vi "Run.vi"(8 "error in (no error)":errorcluster, 11 "Channel in":refnum<class "Channel.lvclass">) -> (0 "error out":errorcluster, 3 "Channel out":refnum<class "Channel.lvclass">)   [LabVIEW 2018, in "Channel.lvclass"]
uses:
  Channel.lvclass
  Channel.lvclass/Channel.ctl
  Simulated_CCD_Camera/Simulated_CCD_Camera.lvclass/Simulated_CCD_Camera.ctl
  State Machine/State Machine.lvclass/State Machine.ctl
  Save Image/Save Image.lvclass/Save Image.ctl
  Interface/Interface.lvclass/Interface.ctl
  Interface/Interface.lvclass
  State Machine/State Machine.lvclass
  Simulated_CCD_Camera/Simulated_CCD_Camera.lvclass
  Save Image/Save Image.lvclass
  RxTx/RxTx.lvclass
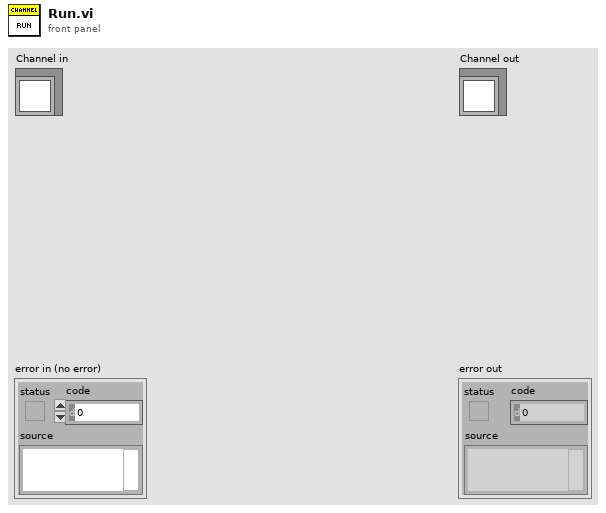
[diagram p1: front panel]
types:
  T1 = cluster{"PREAMP":u16, "READOUT_RATE":u16, "EM_GAIN":u16, "VBIN":u16, "INITIAL_LINE":u16, "INITIAL_COLUMN":u16, "FINAL_LINE":u16, "FINAL_COLUMN":u16, "TRIGGER_MODE":u16, "HBIN":u16, "SHUTTER_TTL":u16, "SHUTTER_MODE":u16, "SHUTTER_OPENING_TIME":u16, "SHUTTER_CLOSING_TIME":u16, "VERTICAL_SHIFT_SPEED":u16, "READ_MODE":u16, "FRAME_TRANSFER":bool, "VERTICAL_CLOCK_VOLTAGE":u16, "ACQUISITION_MODE":u16, "AD_CHANNEL":u16, "EM_MODE":u16}
  T2 = cluster{"CUBE_EXPOSURE_TIME":sgl, "CUBES_DONE":u16, "LAST_IMAGE_NAME":string, "DISK_SPACE":u16, "FRAMES_DONE":u16, "CCD_STATUS":string, "CURRENT_TEMPERATURE":i16, "TEMPERATURE_STATUS":string, "FRAME_EXPOSURE_TIME":u16, "CCD_ON_OFF":bool, "SERIAL_NUMBER":u16, "ACQUIRING":bool}
  T3 = typedef "Shutter_mode typedef.ctl" = enum16{"Auto", "Open", "Close", "N/A (3)", "Open FVB Series", "Open Any Series"}
  T4 = typedef "ReadMode_mode typedef.ctl" = enum16{"Full Vertical Binning", "Multi-Track", "Random-Track", "Single-Track", "Image"}
  T5 = typedef "AcquisitionMode_mode typedef.ctl" = enum16{"Reserved (0)", "Single Scan", "Accumulate", "Kinetics", "Fast Kinetics", "Run Till Abort", "Reserved (6)", "Reserved (7)", "Reserved (8)", "Time Delayed Integration"}
  T6 = cluster{"PREAMP":enum16{"Gain 1", "Gain 2"}, "READOUT_RATE":enum16{"30 MHz", "20 MHz", "10 MHz", "1 MHz"}, "EM_GAIN":u16, "VBIN":u16, "INITIAL_LINE":u16, "INITIAL_COLUMN":u16, "FINAL_LINE":u16, "FINAL_COLUMN":u16, "TRIGGER_MODE":enum16{"Internal", "External", "N/A", "N/A_1", "N/A_2", "N/A_3", "External Start"}, "HBIN":u16, "SHUTTER_TTL":enum16{"TTL Low", "TTL High"}, "SHUTTER_MODE":T3, "SHUTTER_OPENING_TIME":u16, "SHUTTER_CLOSING_TIME":u16, "VERTICAL_SHIFT_SPEED":u16, "READ_MODE":T4, "FRAME_TRANSFER":bool, "VERTICAL_CLOCK_VOLTAGE":enum16{"0", "+1", "+2", "+3", "+4"}, "ACQUISITION_MODE":T5, "AD_CHANNEL":u16, "EM_MODE":enum16{"Electron Multiplying", "Conventional"}}
  T7 = cluster{"COMNENT":string, "OBSTYPE":string, "ACSVRSN":string, "CHANNEL":u16, "LAST_IMG_NAME":string, "NIGHTDIR":string}
  T8 = cluster{"COOLER_POWER_STATUS":u16, "TEMP":i32, "EXPTIME":dbl, "#FRAMES":u32, "#CUBES":u32}
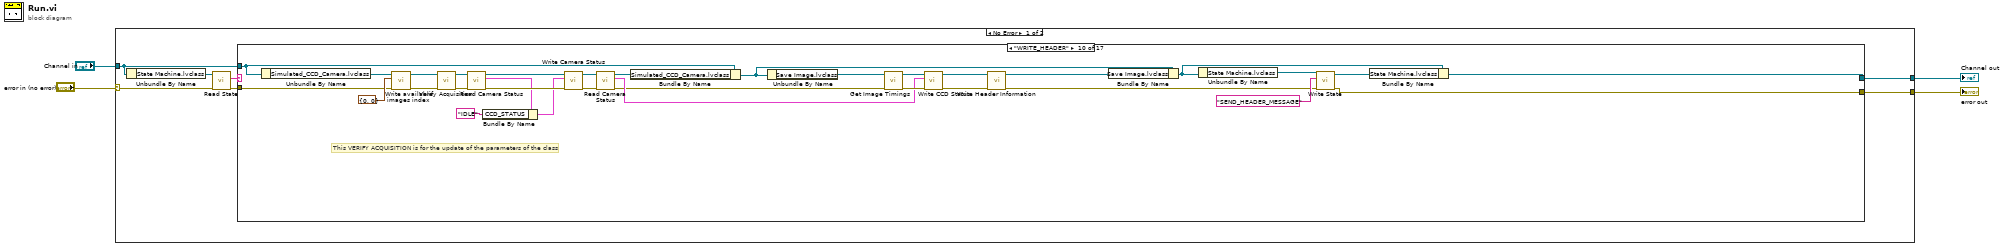
[diagram p0: block diagram]
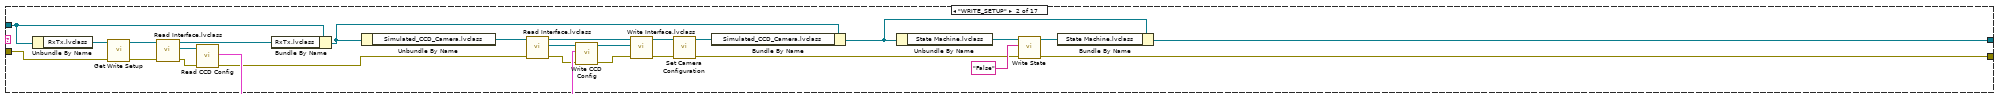
[diagram p3: hidden frame]
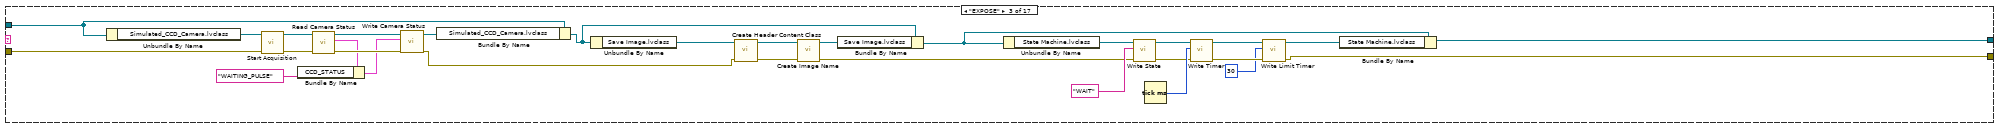
[diagram p4: hidden frame]
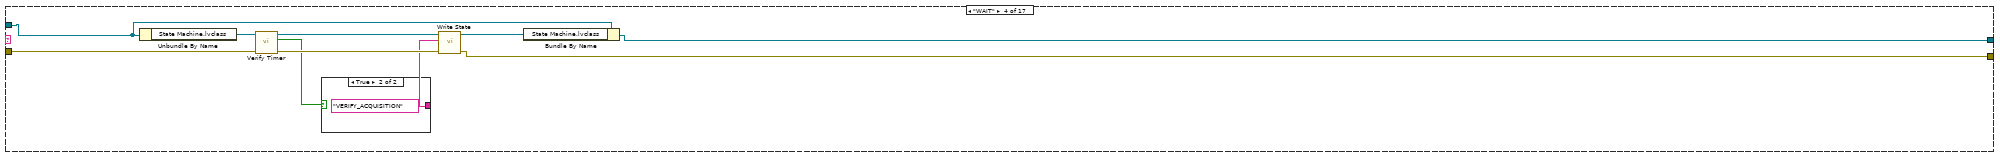
[diagram p5: hidden frame]
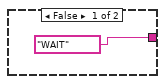
[diagram p6: hidden frame]
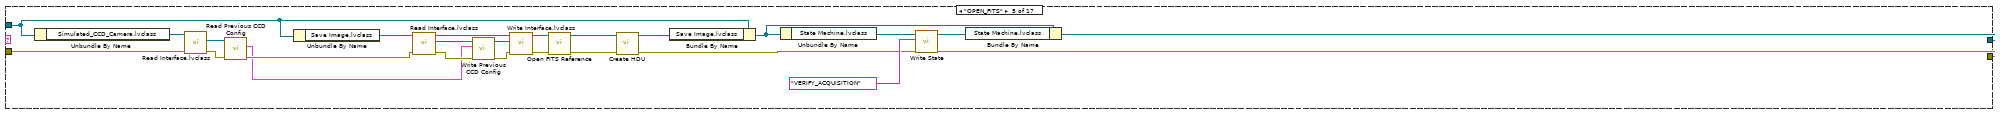
[diagram p7: hidden frame]
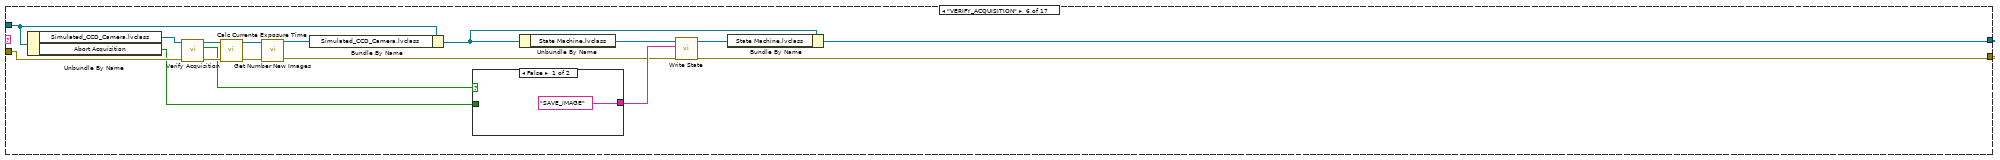
[diagram p8: hidden frame]
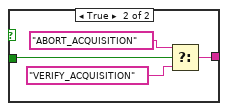
[diagram p9: hidden frame]
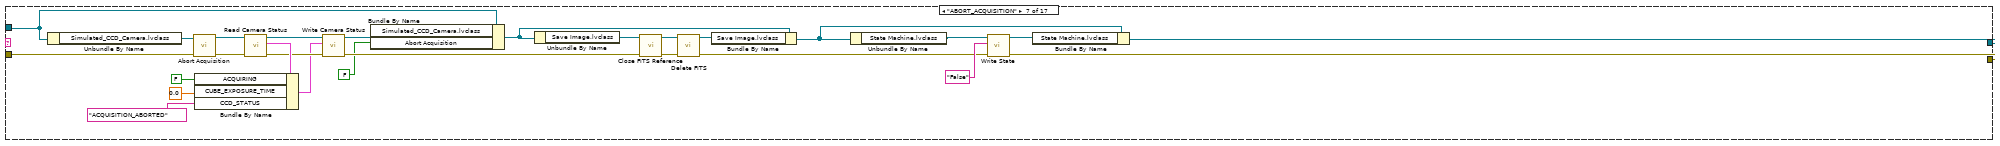
[diagram p10: hidden frame]
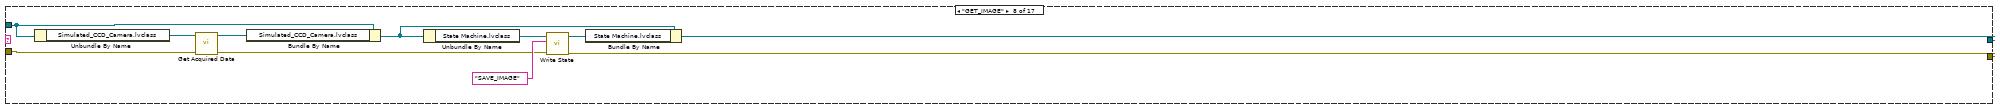
[diagram p11: hidden frame]
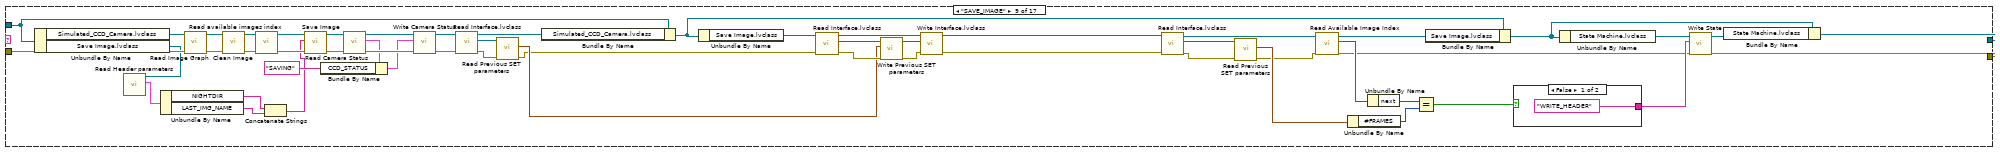
[diagram p12: hidden frame]
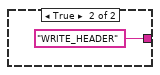
[diagram p13: hidden frame]
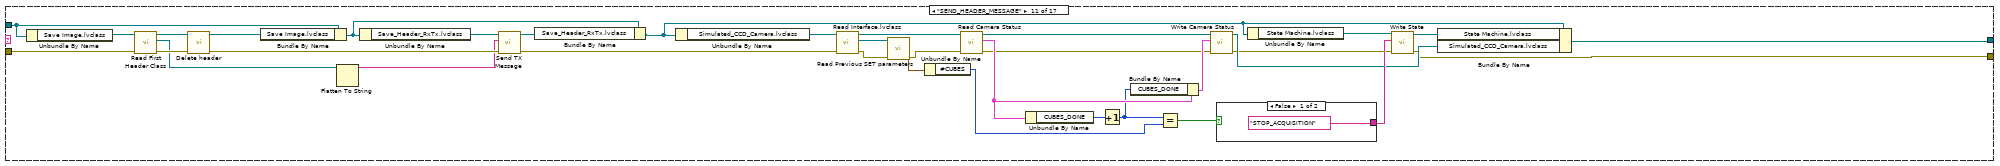
[diagram p14: hidden frame]
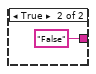
[diagram p15: hidden frame]
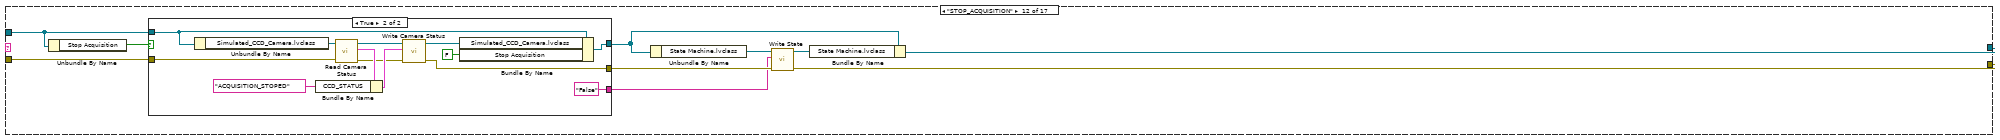
[diagram p16: hidden frame]
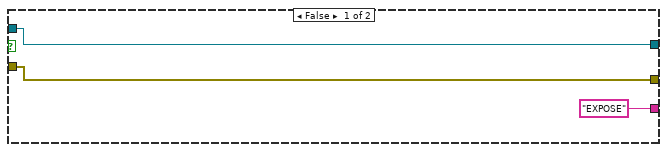
[diagram p17: hidden frame]
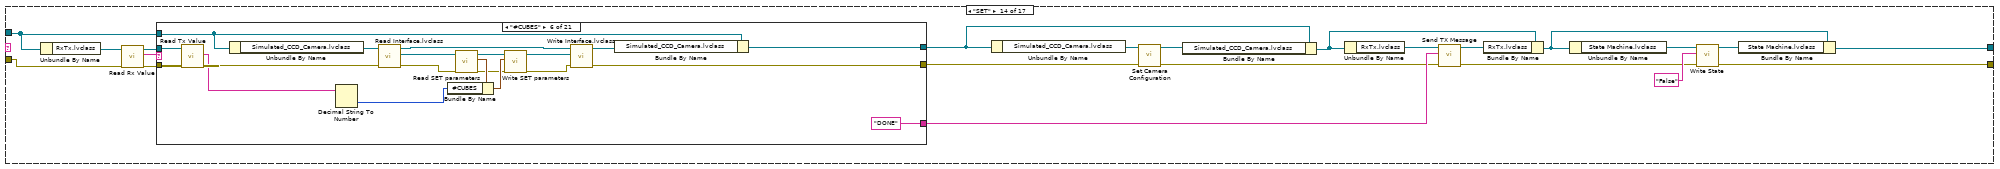
[diagram p19: hidden frame]
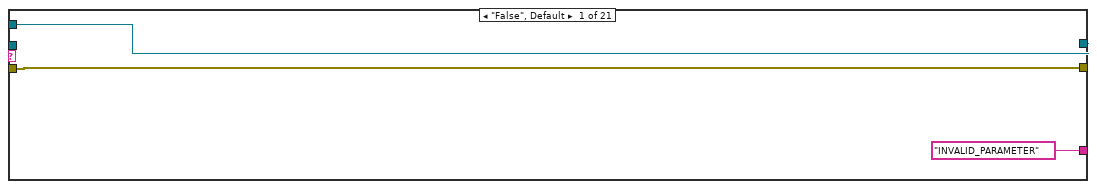
[diagram p20: hidden frame]
diagram:
  n1 = case shown="No Error" "error in (no error)" {
    selector: "error in (no error)" -> [w7 w973]
    tunnel: [w11 w973] -> w3
    tunnel: [w9 w972] -> w1
    tunnel: "Channel in" -> [w10 w972]
    frame No Error {
      n2 = Unbundle By Name(w10) -> ("State Machine.lvclass"=w8:refnum<class "State Machine.lvclass">)
      n3 = call-dynamic "Read State.vi"("error in (no error)"=w7, "State Machine in"=w8) -> ("error out"=w6:errorcluster, "State"=w5:string)  [unwired: 7 in, 1 out]
      n4 = case shown="\"WRITE_HEADER\"" w5 {
        tunnel: w6 -> [w12 w33 w57 w79 w99 w110 w136 w159 w201 w231 w272 w298 w319 w334 w737 w912 w945]
        tunnel: [w12 w28 w46 w71 w104 w119 w152 w162 w211 w233 w277 w299 w319 w321 w730 w932 w938] -> w11
        tunnel: [w13 w29 w60 w72 w107 w122 w155 w167 w212 w243 w287 w302 w320 w322 w731 w933 w939] -> w9
        tunnel: w10 -> [w13 w34 w55 w76 w101 w124 w135 w166 w199 w230 w276 w295 w320 w335 w738 w925 w944]
        frame "False", Default {
        }
        frame "WRITE_SETUP" {
          n5 = Unbundle By Name(w34) -> ("RxTx.lvclass"=w36:refnum<class "RxTx.lvclass">)
          n6 = call "Get Write Setup.vi"("error in (no error)"=w33, "RxTx in"=w36) -> ("error out"=w37:errorcluster, "RxTx out"=w38:refnum<class "RxTx.lvclass">)  [unwired: 8 in]
          n7 = call "Read Interface.lvclass.vi"("error in (no error)"=w37, "RxTx in"=w38) -> ("error out"=w21:errorcluster, "Interface.lvclass"=w22:refnum<class "Interface.lvclass">, "RxTx out"=w39:refnum<class "RxTx.lvclass">)  [unwired: 7 in]
          n8 = call "Read CCD Config.vi"("error in (no error)"=w21, "Interface in"=w22) -> ("error out"=w15:errorcluster, "Previous CCD Config"=w20:T1)  [unwired: 7 in, 1 out]
          n9 = Bundle By Name(cluster=w34, "RxTx.lvclass"=w39) -> (w35:refnum<class "Channel.lvclass">)
          n10 = Unbundle By Name(w35) -> ("Simulated_CCD_Camera.lvclass"=w26:refnum<class "Simulated_CCD_Camera.lvclass">)
          n11 = call "Read Interface.lvclass.vi"("error in (no error)"=w15, "Simulated_CCD_Camera in"=w26) -> ("error out"=w17:errorcluster, "Interface.lvclass"=w18:refnum<class "Interface.lvclass">, "Simulated_CCD_Camera out"=w23:refnum<class "Simulated_CCD_Camera.lvclass">)  [unwired: 7 in]
          n12 = call "Write CCD Config.vi"("error in (no error)"=w17, "CCD Config"=w20, "Interface in"=w18) -> ("error out"=w16:errorcluster, "Interface out"=w19:refnum<class "Interface.lvclass">)  [unwired: 7 in]
          n13 = call "Write Interface.lvclass.vi"("error in (no error)"=w16, "Interface.lvclass"=w19, "Simulated_CCD_Camera in"=w23) -> ("error out"=w24:errorcluster, "Simulated_CCD_Camera out"=w25:refnum<class "Simulated_CCD_Camera.lvclass">)  [unwired: 7 in]
          n14 = call-dynamic "Set Camera Configuration.vi"("error in (no error)"=w24, "CCDCamera in"=w25) -> ("error out"=w27:errorcluster, "CCDCamera out"=w14:refnum<class "Simulated_CCD_Camera.lvclass">)  [unwired: 8 in]
          n15 = Bundle By Name(cluster=w35, "Simulated_CCD_Camera.lvclass"=w14) -> (w40:refnum<class "Channel.lvclass">)
          n16 = Unbundle By Name(w40) -> ("State Machine.lvclass"=w31:refnum<class "State Machine.lvclass">)
          n17 = call-dynamic "Write State.vi"("error in (no error)"=w27, "State"="False", "State Machine in"=w31) -> ("error out"=w28:errorcluster, "State Machine out"=w32:refnum<class "State Machine.lvclass">)  [unwired: 7 in]
          n18 = Bundle By Name(cluster=w40, "State Machine.lvclass"=w32) -> (w29:refnum<class "Channel.lvclass">)
        }
        frame "EXPOSE" {
          n19 = Unbundle By Name(w55) -> ("Simulated_CCD_Camera.lvclass"=w58:refnum<class "Simulated_CCD_Camera.lvclass">)
          n20 = call-dynamic "Start Acquisition.vi"("error in (no error)"=w57, "CCDCamera in"=w58) -> ("error out"=w69:errorcluster, "CCDCamera out"=w70:refnum<class "Simulated_CCD_Camera.lvclass">)  [unwired: 8 in]
          n21 = call "Read Camera Status.vi"("error in (no error)"=w69, "CCDCamera in"=w70) -> ("error out"=w67:errorcluster, "Camera Status"=w66:T2, "CCDCamera out"=w68:refnum<class "Simulated_CCD_Camera.lvclass">)  [unwired: 7 in]
          n22 = Bundle By Name(cluster=w66, "CCD_STATUS"="WAITING_PULSE" ("STATUS")) -> (w64:T2)
          n23 = call "Write Camera Status.vi"("error in (no error)"=w67, "Camera Status"=w64, "CCDCamera in"=w68) -> ("error out"=w42:errorcluster, "CCDCamera out"=w54:refnum<class "Simulated_CCD_Camera.lvclass">)  [unwired: 7 in]
          n24 = Bundle By Name(cluster=w55, "Simulated_CCD_Camera.lvclass"=w54) -> (w53:refnum<class "Channel.lvclass">)
          n25 = Unbundle By Name(w53) -> ("Save Image.lvclass"=w41:refnum<class "Save Image.lvclass">)
          n26 = call "Create Header Content Class.vi"("error in (no error)"=w42, "Save Image in"=w41) -> ("error out"=w43:errorcluster, "Save Image out"=w44:refnum<class "Save Image.lvclass">)  [unwired: 8 in]
          n27 = call "Create Image Name.vi"("error in (no error)"=w43, "Save Image in"=w44) -> ("error out"=w56:errorcluster, "Save Image out"=w59:refnum<class "Save Image.lvclass">)  [unwired: 8 in]
          n28 = Bundle By Name(cluster=w53, "Save Image.lvclass"=w59) -> (w61:refnum<class "Channel.lvclass">)
          n29 = Unbundle By Name(w61) -> ("State Machine.lvclass"=w65:refnum<class "State Machine.lvclass">)
          n30 = call-dynamic "Write State.vi"("error in (no error)"=w56, "State"="WAIT", "State Machine in"=w65) -> ("error out"=w50:errorcluster, "State Machine out"=w51:refnum<class "State Machine.lvclass">)  [unwired: 7 in]
          n31 = Tick Count (ms)() -> (millisecond timer value=w52:u32)
          n32 = call "Write Timer.vi"("error in (no error)"=w50, "Timer"=w52, "State Machine in"=w51) -> ("error out"=w47:errorcluster, "State Machine out"=w49:refnum<class "State Machine.lvclass">)  [unwired: 7 in]
          n33 = call "Write Limit Timer.vi"("error in (no error)"=w47, "Limit Timer"=30, "State Machine in"=w49) -> ("error out"=w46:errorcluster, "State Machine out"=w48:refnum<class "State Machine.lvclass">)  [unwired: 7 in]
          n34 = Bundle By Name(cluster=w61, "State Machine.lvclass"=w48) -> (w60:refnum<class "Channel.lvclass">)
        }
        frame "WAIT" {
          n35 = Unbundle By Name(w76) -> ("State Machine.lvclass"=w80:refnum<class "State Machine.lvclass">)
          n36 = call "Verify Timer.vi"("error in (no error)"=w79, "State Machine in"=w80) -> ("error out"=w77:errorcluster, "time out"=w74:bool, "State Machine out"=w78:refnum<class "State Machine.lvclass">)  [unwired: 7 in]
          n37 = case shown="True" w74 {
            tunnel: ["WAIT" "VERIFY_ACQUISITION"] -> w73
            frame False {
            }
            frame True {
            }
          }
          n38 = call-dynamic "Write State.vi"("error in (no error)"=w77, "State"=w73, "State Machine in"=w78) -> ("error out"=w71:errorcluster, "State Machine out"=w75:refnum<class "State Machine.lvclass">)  [unwired: 7 in]
          n39 = Bundle By Name(cluster=w76, "State Machine.lvclass"=w75) -> (w72:refnum<class "Channel.lvclass">)
        }
        frame "OPEN_FITS" {
          n40 = Unbundle By Name(w101) -> ("Simulated_CCD_Camera.lvclass"=w100:refnum<class "Simulated_CCD_Camera.lvclass">)
          n41 = call "Read Interface.lvclass.vi"("error in (no error)"=w99, "Simulated_CCD_Camera in"=w100) -> ("error out"=w97:errorcluster, "Interface.lvclass"=w98:refnum<class "Interface.lvclass">)  [unwired: 7 in, 1 out]
          n42 = call "Read Previous CCD Config.vi"("error in (no error)"=w97, "Interface in"=w98) -> ("error out"=w88:errorcluster, "Previous CCD Config"=w87:T6)  [unwired: 7 in, 1 out]
          n43 = Unbundle By Name(w101) -> ("Save Image.lvclass"=w91:refnum<class "Save Image.lvclass">)
          n44 = call "Read Interface.lvclass.vi"("error in (no error)"=w88, "Save Image in"=w91) -> ("error out"=w92:errorcluster, "Interface.lvclass"=w96:refnum<class "Interface.lvclass">, "Save Image out"=w94:refnum<class "Save Image.lvclass">)  [unwired: 7 in]
          n45 = call "Write Previous CCD Config.vi"("error in (no error)"=w92, "Previous CCD Config"=w87, "Interface in"=w96) -> ("error out"=w93:errorcluster, "Interface out"=w95:refnum<class "Interface.lvclass">)  [unwired: 7 in]
          n46 = call "Write Interface.lvclass.vi"("error in (no error)"=w93, "Interface.lvclass"=w95, "Save Image in"=w94) -> ("error out"=w89:errorcluster, "Save Image out"=w90:refnum<class "Save Image.lvclass">)  [unwired: 7 in]
          n47 = call "Open FITS Reference.vi"("error in (no error)"=w89, "Save Image in"=w90) -> ("error out"=w84:errorcluster, "Save Image out"=w86:refnum<class "Save Image.lvclass">)  [unwired: 8 in]
          n48 = call "Create HDU.vi"("error in (no error)"=w84, "Save Image in"=w86) -> ("error out"=w83:errorcluster, "Save Image out"=w85:refnum<class "Save Image.lvclass">)  [unwired: 8 in]
          n49 = Bundle By Name(cluster=w101, "Save Image.lvclass"=w85) -> (w103:refnum<class "Channel.lvclass">)
          n50 = Unbundle By Name(w103) -> ("State Machine.lvclass"=w105:refnum<class "State Machine.lvclass">)
          n51 = call-dynamic "Write State.vi"("error in (no error)"=w83, "State"="VERIFY_ACQUISITION", "State Machine in"=w105) -> ("error out"=w104:errorcluster, "State Machine out"=w106:refnum<class "State Machine.lvclass">)  [unwired: 7 in]
          n52 = Bundle By Name(cluster=w103, "State Machine.lvclass"=w106) -> (w107:refnum<class "Channel.lvclass">)
        }
        frame "VERIFY_ACQUISITION" {
          n53 = Unbundle By Name(w124) -> ("Simulated_CCD_Camera.lvclass"=w111:refnum<class "Simulated_CCD_Camera.lvclass">, "Abort Acquisition"=w109:bool)
          n54 = call-dynamic "Verify Acquisition.vi"("error in (no error)"=w110, "CCDCamera in"=w111) -> ("error out"=w114:errorcluster, "Acquiring"=w108:bool, "CCDCamera out"=w115:refnum<class "Simulated_CCD_Camera.lvclass">)  [unwired: 7 in]
          n55 = call-dynamic "Calc Currente Exposure Time.vi"("error in (no error)"=w114, "CCDCamera in"=w115) -> ("error out"=w116:errorcluster, "CCDCamera out"=w117:refnum<class "Simulated_CCD_Camera.lvclass">)  [unwired: 8 in]
          n56 = call-dynamic "Get Number New Images.vi"("error in (no error)"=w116, "CCDCamera in"=w117) -> ("error out"=w112:errorcluster, "CCDCamera out"=w113:refnum<class "Simulated_CCD_Camera.lvclass">)  [unwired: 7 in, 1 out]
          n57 = Bundle By Name(cluster=w124, "Simulated_CCD_Camera.lvclass"=w113) -> (w123:refnum<class "Channel.lvclass">)
          n58 = case shown="False" w108 {
            tunnel: ["SAVE_IMAGE" w127] -> w118
            tunnel: w109 -> [_ w126]
            frame False {
            }
            frame True {
              n59 = Select(t="ABORT_ACQUISITION", s=w126, f="VERIFY_ACQUISITION") -> (s? t:f=w127:string)
            }
          }
          n60 = Unbundle By Name(w123) -> ("State Machine.lvclass"=w121:refnum<class "State Machine.lvclass">)
          n61 = call-dynamic "Write State.vi"("error in (no error)"=w112, "State"=w118, "State Machine in"=w121) -> ("error out"=w119:errorcluster, "State Machine out"=w120:refnum<class "State Machine.lvclass">)  [unwired: 7 in]
          n62 = Bundle By Name(cluster=w123, "State Machine.lvclass"=w120) -> (w122:refnum<class "Channel.lvclass">)
        }
        frame "ABORT_ACQUISITION" {
          n63 = Unbundle By Name(w135) -> ("Simulated_CCD_Camera.lvclass"=w137:refnum<class "Simulated_CCD_Camera.lvclass">)
          n64 = call-dynamic "Abort Acquisition.vi"("error in (no error)"=w136, "CCDCamera in"=w137) -> ("error out"=w146:errorcluster, "CCDCamera out"=w147:refnum<class "Simulated_CCD_Camera.lvclass">)  [unwired: 8 in]
          n65 = call "Read Camera Status.vi"("error in (no error)"=w146, "CCDCamera in"=w147) -> ("error out"=w144:errorcluster, "Camera Status"=w150:T2, "CCDCamera out"=w145:refnum<class "Simulated_CCD_Camera.lvclass">)  [unwired: 7 in]
          n66 = Bundle By Name(cluster=w150, "ACQUIRING"=FALSE ("Acquiring"), "CUBE_EXPOSURE_TIME"=sgl 0.0 ("Current exptime"), "CCD_STATUS"="ACQUISITION_ABORTED" ("STATUS")) -> (w143:T2)
          n67 = call "Write Camera Status.vi"("error in (no error)"=w144, "Camera Status"=w143, "CCDCamera in"=w145) -> ("error out"=w132:errorcluster, "CCDCamera out"=w134:refnum<class "Simulated_CCD_Camera.lvclass">)  [unwired: 7 in]
          n68 = Bundle By Name(cluster=w135, "Simulated_CCD_Camera.lvclass"=w134, "Abort Acquisition"=FALSE ("Acquiring")) -> (w131:refnum<class "Channel.lvclass">)
          n69 = Unbundle By Name(w131) -> ("Save Image.lvclass"=w133:refnum<class "Save Image.lvclass">)
          n70 = call "Close FITS Reference.vi"("error in (no error)"=w132, "Save Image in"=w133) -> ("error out"=w141:errorcluster, "Save Image out"=w142:refnum<class "Save Image.lvclass">)  [unwired: 8 in]
          n71 = call "Delete FITS.vi"("error in (no error)"=w141, "Save Image in"=w142) -> ("error out"=w138:errorcluster, "Save Image out"=w139:refnum<class "Save Image.lvclass">)  [unwired: 8 in]
          n72 = Bundle By Name(cluster=w131, "Save Image.lvclass"=w139) -> (w156:refnum<class "Channel.lvclass">)
          n73 = Unbundle By Name(w156) -> ("State Machine.lvclass"=w154:refnum<class "State Machine.lvclass">)
          n74 = call-dynamic "Write State.vi"("error in (no error)"=w138, "State"="False", "State Machine in"=w154) -> ("error out"=w152:errorcluster, "State Machine out"=w153:refnum<class "State Machine.lvclass">)  [unwired: 7 in]
          n75 = Bundle By Name(cluster=w156, "State Machine.lvclass"=w153) -> (w155:refnum<class "Channel.lvclass">)
        }
        frame "GET_IMAGE" {
          n76 = Unbundle By Name(w166) -> ("Simulated_CCD_Camera.lvclass"=w160:refnum<class "Simulated_CCD_Camera.lvclass">)
          n77 = call-dynamic "Get Acquired Data.vi"("error in (no error)"=w159, "CCDCamera in"=w160) -> ("error out"=w157:errorcluster, "CCDCamera out"=w158:refnum<class "Simulated_CCD_Camera.lvclass">)  [unwired: 8 in]
          n78 = Bundle By Name(cluster=w166, "Simulated_CCD_Camera.lvclass"=w158) -> (w165:refnum<class "Channel.lvclass">)
          n79 = Unbundle By Name(w165) -> ("State Machine.lvclass"=w163:refnum<class "State Machine.lvclass">)
          n80 = call-dynamic "Write State.vi"("error in (no error)"=w157, "State"="SAVE_IMAGE", "State Machine in"=w163) -> ("error out"=w162:errorcluster, "State Machine out"=w164:refnum<class "State Machine.lvclass">)  [unwired: 7 in]
          n81 = Bundle By Name(cluster=w165, "State Machine.lvclass"=w164) -> (w167:refnum<class "Channel.lvclass">)
        }
        frame "SAVE_IMAGE" {
          n82 = Unbundle By Name(w199) -> ("Simulated_CCD_Camera.lvclass"=w200:refnum<class "Simulated_CCD_Camera.lvclass">, "Save Image.lvclass"=w172:refnum<class "Save Image.lvclass">)
          n83 = call "Read Header parameters.vi"("Save Image in"=w172) -> ("Header parameters"=w171:T7)  [unwired: 8 in, 2 out]
          n84 = Unbundle By Name(w171) -> ("NIGHTDIR"=w170:string, "LAST_IMG_NAME"=w169:string)
          n85 = call "Read Image Graph.vi"("error in (no error)"=w201, "CCDCamera in"=w200) -> ("error out"=w220:errorcluster, "CCDCamera out"=w221:refnum<class "Simulated_CCD_Camera.lvclass">)  [unwired: 7 in, 1 out]
          n86 = call "Clean Image.vi"("error in (no error)"=w220, "CCDCamera in"=w221) -> ("error out"=w218:errorcluster, "CCDCamera out"=w219:refnum<class "Simulated_CCD_Camera.lvclass">)  [unwired: 8 in]
          n87 = call "Read available images index.vi"("error in (no error)"=w218, "CCDCamera in"=w219) -> ("error out"=w174:errorcluster, "CCDCamera out"=w173:refnum<class "Simulated_CCD_Camera.lvclass">)  [unwired: 7 in, 1 out]
          n88 = Concatenate Strings(w170, w169) -> (w168:string)
          n89 = call-dynamic "Save Image.vi"("error in (no error)"=w174, "path"=w168, "Simulated_CCD_Camera in"=w173) -> ("error out"=w175:errorcluster, "Simulated_CCD_Camera out"=w176:refnum<class "Simulated_CCD_Camera.lvclass">)  [unwired: 7 in]
          n90 = call "Read Camera Status.vi"("error in (no error)"=w175, "CCDCamera in"=w176) -> ("error out"=w208:errorcluster, "Camera Status"=w205:T2, "CCDCamera out"=w206:refnum<class "Simulated_CCD_Camera.lvclass">)  [unwired: 7 in]
          n91 = Bundle By Name(cluster=w205, "CCD_STATUS"="SAVING" ("STATUS")) -> (w204:T2)
          n92 = call "Write Camera Status.vi"("error in (no error)"=w208, "Camera Status"=w204, "CCDCamera in"=w206) -> ("error out"=w190:errorcluster, "CCDCamera out"=w191:refnum<class "Simulated_CCD_Camera.lvclass">)  [unwired: 7 in]
          n93 = call "Read Interface.lvclass.vi"("error in (no error)"=w190, "Simulated_CCD_Camera in"=w191) -> ("error out"=w187:errorcluster, "Interface.lvclass"=w188:refnum<class "Interface.lvclass">, "Simulated_CCD_Camera out"=w189:refnum<class "Simulated_CCD_Camera.lvclass">)  [unwired: 7 in]
          n94 = call "Read Previous SET parameters.vi"("error in (no error)"=w187, "Interface in"=w188) -> ("error out"=w177:errorcluster, "Previous SET parameters"=w178:T8)  [unwired: 7 in, 1 out]
          n95 = Bundle By Name(cluster=w199, "Simulated_CCD_Camera.lvclass"=w189) -> (w198:refnum<class "Channel.lvclass">)
          n96 = Unbundle By Name(w198) -> ("Save Image.lvclass"=w181:refnum<class "Save Image.lvclass">)
          n97 = call "Read Interface.lvclass.vi"("error in (no error)"=w177, "Save Image in"=w181) -> ("error out"=w183:errorcluster, "Interface.lvclass"=w184:refnum<class "Interface.lvclass">, "Save Image out"=w182:refnum<class "Save Image.lvclass">)  [unwired: 7 in]
          n98 = call "Write Previous SET parameters.vi"("error in (no error)"=w183, "Previous SET parameters"=w178, "Interface in"=w184) -> ("error out"=w185:errorcluster, "Interface out"=w186:refnum<class "Interface.lvclass">)  [unwired: 7 in]
          n99 = call "Write Interface.lvclass.vi"("error in (no error)"=w185, "Interface.lvclass"=w186, "Save Image in"=w182) -> ("error out"=w179:errorcluster, "Save Image out"=w180:refnum<class "Save Image.lvclass">)  [unwired: 7 in]
          n100 = call "Read Interface.lvclass.vi"("error in (no error)"=w179, "Save Image in"=w180) -> ("error out"=w192:errorcluster, "Interface.lvclass"=w194:refnum<class "Interface.lvclass">, "Save Image out"=w197:refnum<class "Save Image.lvclass">)  [unwired: 7 in]
          n101 = call "Read Previous SET parameters.vi"("error in (no error)"=w192, "Interface in"=w194) -> ("error out"=w193:errorcluster, "Previous SET parameters"=w196:T8)  [unwired: 7 in, 1 out]
          n102 = call "Read Available Image Index.vi"("error in (no error)"=w193, "Save Image in"=w197) -> ("error out"=w202:errorcluster, "available images index"=w210:cluster{"previous":u16, "next":u16}, "Save Image out"=w203:refnum<class "Save Image.lvclass">)  [unwired: 7 in]
          n103 = Unbundle By Name(w196) -> ("#FRAMES"=w195:u32)
          n104 = Unbundle By Name(w210) -> ("next"=w209:u16)
          n105 = Equal?(x=w209, y=w195) -> (x = y?=w217:bool)
          n106 = Bundle By Name(cluster=w198, "Save Image.lvclass"=w203) -> (w214:refnum<class "Channel.lvclass">)
          n107 = case shown="False" w217 {
            tunnel: ["WRITE_HEADER" "WRITE_HEADER"] -> w215
            frame False {
            }
            frame True {
            }
          }
          n108 = Unbundle By Name(w214) -> ("State Machine.lvclass"=w216:refnum<class "State Machine.lvclass">)
          n109 = call-dynamic "Write State.vi"("error in (no error)"=w202, "State"=w215, "State Machine in"=w216) -> ("error out"=w211:errorcluster, "State Machine out"=w213:refnum<class "State Machine.lvclass">)  [unwired: 7 in]
          n110 = Bundle By Name(cluster=w214, "State Machine.lvclass"=w213) -> (w212:refnum<class "Channel.lvclass">)
        }
        frame "WRITE_HEADER" {
          # "This VERIFY ACQUISITION is for the update of the parameters of the class"
          n111 = Unbundle By Name(w230) -> ("Simulated_CCD_Camera.lvclass"=w232:refnum<class "Simulated_CCD_Camera.lvclass">)
          n112 = call "Write available images index.vi"("error in (no error)"=w231, "available images index"=cluster{"previous":u16, "next":u16} {"previous"=0, "next"=0}, "CCDCamera in"=w232) -> ("error out"=w253:errorcluster, "CCDCamera out"=w254:refnum<class "Simulated_CCD_Camera.lvclass">)  [unwired: 7 in]
          n113 = call-dynamic "Verify Acquisition.vi"("error in (no error)"=w253, "CCDCamera in"=w254) -> ("error out"=w247:errorcluster, "CCDCamera out"=w248:refnum<class "Simulated_CCD_Camera.lvclass">)  [unwired: 7 in, 1 out]
          n114 = call "Read Camera Status.vi"("error in (no error)"=w247, "CCDCamera in"=w248) -> ("error out"=w251:errorcluster, "Camera Status"=w250:T2, "CCDCamera out"=w252:refnum<class "Simulated_CCD_Camera.lvclass">)  [unwired: 7 in]
          n115 = Bundle By Name(cluster=w250, "CCD_STATUS"="IDLE" ("STATUS")) -> (w249:T2)
          n116 = call "Write Camera Status.vi"("error in (no error)"=w251, "Camera Status"=w249, "CCDCamera in"=w252) -> ("error out"=w241:errorcluster, "CCDCamera out"=w242:refnum<class "Simulated_CCD_Camera.lvclass">)  [unwired: 7 in]
          n117 = call "Read Camera Status.vi"("error in (no error)"=w241, "CCDCamera in"=w242) -> ("error out"=w227:errorcluster, "Camera Status"=w238:T2, "CCDCamera out"=w229:refnum<class "Simulated_CCD_Camera.lvclass">)  [unwired: 7 in]
          n118 = Bundle By Name(cluster=w230, "Simulated_CCD_Camera.lvclass"=w229) -> (w226:refnum<class "Channel.lvclass">)
          n119 = Unbundle By Name(w226) -> ("Save Image.lvclass"=w228:refnum<class "Save Image.lvclass">)
          n120 = call "Get Image Timings.vi"("error in (no error)"=w227, "Save Image in"=w228) -> ("error out"=w239:errorcluster, "Save Image out"=w240:refnum<class "Save Image.lvclass">)  [unwired: 8 in]
          n121 = call "Write CCD Status.vi"("error in (no error)"=w239, "Camera Status"=w238, "Save Image in"=w240) -> ("error out"=w236:errorcluster, "Save Image out"=w237:refnum<class "Save Image.lvclass">)  [unwired: 7 in]
          n122 = call "Write Header Information.vi"("error in (no error)"=w236, "Save Image in"=w237) -> ("error out"=w224:errorcluster, "Save Image out"=w225:refnum<class "Save Image.lvclass">)  [unwired: 8 in]
          n123 = Bundle By Name(cluster=w226, "Save Image.lvclass"=w225) -> (w235:refnum<class "Channel.lvclass">)
          n124 = Unbundle By Name(w235) -> ("State Machine.lvclass"=w234:refnum<class "State Machine.lvclass">)
          n125 = call-dynamic "Write State.vi"("error in (no error)"=w224, "State"="SEND_HEADER_MESSAGE", "State Machine in"=w234) -> ("error out"=w233:errorcluster, "State Machine out"=w245:refnum<class "State Machine.lvclass">)  [unwired: 7 in]
          n126 = Bundle By Name(cluster=w235, "State Machine.lvclass"=w245) -> (w243:refnum<class "Channel.lvclass">)
        }
        frame "SEND_HEADER_MESSAGE" {
          n127 = Unbundle By Name(w276) -> ("Save Image.lvclass"=w273:refnum<class "Save Image.lvclass">)
          n128 = call "Read First Header Class.vi"("error in (no error)"=w272, "Save Image in"=w273) -> ("error out"=w269:errorcluster, "Simulated_Header.lvclass"=w266:refnum<class "Simulated_Header.lvclass">, "Save Image out"=w271:refnum<class "Save Image.lvclass">)  [unwired: 7 in]
          n129 = call "Delete header.vi"("error in (no error)"=w269, "Save Image in"=w271) -> ("error out"=w267:errorcluster, "Save Image out"=w270:refnum<class "Save Image.lvclass">)  [unwired: 8 in]
          n130 = Bundle By Name(cluster=w276, "Save Image.lvclass"=w270) -> (w264:refnum<class "Channel.lvclass">)
          n131 = Flatten To String(anything=w266) -> (data string=w265:string)  [unwired: 3 in, 2 out]
          n132 = Unbundle By Name(w264) -> ("Save_Header_RxTx.lvclass"=w268:refnum<class "RxTx.lvclass">)
          n133 = call "Send TX Message.vi"("error in (no error)"=w267, "element"=w265, "RxTx in"=w268) -> ("error out"=w261:errorcluster, "RxTx out"=w263:refnum<class "RxTx.lvclass">)  [unwired: 7 in]
          n134 = Bundle By Name(cluster=w264, "Save_Header_RxTx.lvclass"=w263) -> (w262:refnum<class "Channel.lvclass">)
          n135 = Unbundle By Name(w262) -> ("Simulated_CCD_Camera.lvclass"=w275:refnum<class "Simulated_CCD_Camera.lvclass">)
          n136 = call "Read Interface.lvclass.vi"("error in (no error)"=w261, "Simulated_CCD_Camera in"=w275) -> ("error out"=w257:errorcluster, "Interface.lvclass"=w258:refnum<class "Interface.lvclass">, "Simulated_CCD_Camera out"=w274:refnum<class "Simulated_CCD_Camera.lvclass">)  [unwired: 7 in]
          n137 = call "Read Previous SET parameters.vi"("error in (no error)"=w257, "Interface in"=w258) -> ("error out"=w256:errorcluster, "Previous SET parameters"=w260:T8)  [unwired: 7 in, 1 out]
          n138 = Unbundle By Name(w260) -> ("#CUBES"=w259:u32)
          n139 = call "Read Camera Status.vi"("error in (no error)"=w256, "CCDCamera in"=w274) -> ("error out"=w282:errorcluster, "Camera Status"=w286:T2, "CCDCamera out"=w283:refnum<class "Simulated_CCD_Camera.lvclass">)  [unwired: 7 in]
          n140 = Unbundle By Name(w286) -> ("CUBES_DONE"=w285:u16)
          n141 = Increment(x=w285) -> (x+1=w281:u16)
          n142 = Bundle By Name(cluster=w286, "CUBES_DONE"=w281) -> (w284:T2)
          n143 = Equal?(x=w281, y=w259) -> (x = y?=w288:bool)
          n144 = call "Write Camera Status.vi"("error in (no error)"=w282, "Camera Status"=w284, "CCDCamera in"=w283) -> ("error out"=w279:errorcluster, "CCDCamera out"=w280:refnum<class "Simulated_CCD_Camera.lvclass">)  [unwired: 7 in]
          n145 = case shown="False" w288 {
            tunnel: ["STOP_ACQUISITION" "False"] -> w289
            frame False {
            }
            frame True {
            }
          }
          n146 = Unbundle By Name(w262) -> ("State Machine.lvclass"=w278:refnum<class "State Machine.lvclass">)
          n147 = call-dynamic "Write State.vi"("error in (no error)"=w279, "State"=w289, "State Machine in"=w278) -> ("error out"=w277:errorcluster, "State Machine out"=w290:refnum<class "State Machine.lvclass">)  [unwired: 7 in]
          n148 = Bundle By Name(cluster=w262, "State Machine.lvclass"=w290, "Simulated_CCD_Camera.lvclass"=w280) -> (w287:refnum<class "Channel.lvclass">)
        }
        frame "STOP_ACQUISITION" {
          n149 = Unbundle By Name(w295) -> ("Stop Acquisition"=w294:bool)
          n150 = case shown="True" w294 {
            tunnel: w298 -> [w304 w318]
            tunnel: [w305 w317] -> w297
            tunnel: [w304 w316] -> w296
            tunnel: w295 -> [w305 w308]
            tunnel: ["EXPOSE" "False"] -> w293
            frame False {
            }
            frame True {
              n151 = Unbundle By Name(w308) -> ("Simulated_CCD_Camera.lvclass"=w315:refnum<class "Simulated_CCD_Camera.lvclass">)
              n152 = call "Read Camera Status.vi"("error in (no error)"=w318, "CCDCamera in"=w315) -> ("error out"=w311:errorcluster, "Camera Status"=w313:T2, "CCDCamera out"=w310:refnum<class "Simulated_CCD_Camera.lvclass">)  [unwired: 7 in]
              n153 = Bundle By Name(cluster=w313, "CCD_STATUS"="ACQUISITION_STOPED") -> (w312:T2)
              n154 = call "Write Camera Status.vi"("error in (no error)"=w311, "Camera Status"=w312, "CCDCamera in"=w310) -> ("error out"=w316:errorcluster, "CCDCamera out"=w314:refnum<class "Simulated_CCD_Camera.lvclass">)  [unwired: 7 in]
              n155 = Bundle By Name(cluster=w308, "Simulated_CCD_Camera.lvclass"=w314, "Stop Acquisition"=FALSE) -> (w317:refnum<class "Channel.lvclass">)
            }
          }
          n156 = Unbundle By Name(w297) -> ("State Machine.lvclass"=w301:refnum<class "State Machine.lvclass">)
          n157 = call-dynamic "Write State.vi"("error in (no error)"=w296, "State"=w293, "State Machine in"=w301) -> ("error out"=w299:errorcluster, "State Machine out"=w300:refnum<class "State Machine.lvclass">)  [unwired: 7 in]
          n158 = Bundle By Name(cluster=w297, "State Machine.lvclass"=w300) -> (w302:refnum<class "Channel.lvclass">)
        }
        frame "N/A" {
        }
        frame "SET" {
          n159 = Unbundle By Name(w335) -> ("RxTx.lvclass"=w339:refnum<class "RxTx.lvclass">)
          n160 = call "Read Rx Value.vi"("error in (no error)"=w334, "RxTx in"=w339) -> ("error out"=w341:errorcluster, "Rx value"=w340:string, "RxTx out"=w342:refnum<class "RxTx.lvclass">)  [unwired: 7 in]
          n161 = case shown="\"#CUBES\"" w340 {
            tunnel: [w345 w362 w383 w403 w423 w443 w463 w483 w503 w523 w543 w563 w583 w603 w623 w643 w668 w682 w692 w706 w728] -> w327
            tunnel: w335 -> [w345 w363 w384 w404 w424 w444 w464 w484 w504 w524 w544 w564 w584 w604 w624 w644 w667 w681 w691 w705 w727]
            tunnel: [w344 w359 w381 w401 w421 w441 w461 w481 w501 w521 w541 w561 w581 w601 w621 w641 w658 w671 w683 w695 w718] -> w323
            tunnel: w341 -> [w344 w366 w386 w406 w426 w446 w466 w486 w506 w526 w546 w566 w586 w606 w626 w646 w666 w679 w689 w703 w726]
            tunnel: w342 -> [_ w365 w385 w405 w425 w445 w465 w485 w505 w525 w545 w565 w585 w605 w625 w645 w665 w680 w690 w704 w725]
            tunnel: ["INVALID_PARAMETER" "DONE" "DONE" "DONE" "DONE" "DONE" "DONE" "DONE" "DONE" "DONE" "DONE" "DONE" "DONE" "DONE" "DONE" "DONE" "DONE" "DONE" "DONE" "DONE" "DONE"] -> w336
            frame "False", Default {
            }
            frame "EXPTIME" {
              n162 = call "Read Tx Value.vi"("error in (no error)"=w366, "RxTx in"=w365) -> ("error out"=w356:errorcluster, "Rx Value"=w364:string)  [unwired: 7 in, 1 out]
              n163 = Unbundle By Name(w363) -> ("Simulated_CCD_Camera.lvclass"=w357:refnum<class "Simulated_CCD_Camera.lvclass">)
              n164 = Fract/Exp String To Number(string=w364, default (0 dbl)=sgl 0.0) -> (number=w346:sgl)  [unwired: 2 in, 1 out]
              n165 = call "Read Interface.lvclass.vi"("error in (no error)"=w356, "Simulated_CCD_Camera in"=w357) -> ("error out"=w347:errorcluster, "Interface.lvclass"=w348:refnum<class "Interface.lvclass">, "Simulated_CCD_Camera out"=w355:refnum<class "Simulated_CCD_Camera.lvclass">)  [unwired: 7 in]
              n166 = call "Read SET parameters.vi"("error in (no error)"=w347, "Interface in"=w348) -> ("error out"=w350:errorcluster, "SET parameters"=w353:T8, "Interface out"=w349:refnum<class "Interface.lvclass">)  [unwired: 7 in]
              n167 = Bundle By Name(cluster=w353, "EXPTIME"=w346) -> (w354:T8)
              n168 = call "Write SET parameters.vi"("error in (no error)"=w350, "SET parameters"=w354, "Interface in"=w349) -> ("error out"=w351:errorcluster, "Interface out"=w352:refnum<class "Interface.lvclass">)  [unwired: 7 in]
              n169 = call "Write Interface.lvclass.vi"("error in (no error)"=w351, "Interface.lvclass"=w352, "Simulated_CCD_Camera in"=w355) -> ("error out"=w359:errorcluster, "Simulated_CCD_Camera out"=w358:refnum<class "Simulated_CCD_Camera.lvclass">)  [unwired: 7 in]
              n170 = Bundle By Name(cluster=w363, "Simulated_CCD_Camera.lvclass"=w358) -> (w362:refnum<class "Channel.lvclass">)
            }
            frame "PREAMP" {
              n171 = call "Read Tx Value.vi"("error in (no error)"=w386, "RxTx in"=w385) -> ("error out"=w378:errorcluster, "Rx Value"=w368:string)  [unwired: 7 in, 1 out]
              n172 = Unbundle By Name(w384) -> ("Simulated_CCD_Camera.lvclass"=w379:refnum<class "Simulated_CCD_Camera.lvclass">)
              n173 = Decimal String To Number(string=w368) -> (number=w367:i32)  [unwired: 2 in, 1 out]
              n174 = call "Read Interface.lvclass.vi"("error in (no error)"=w378, "Simulated_CCD_Camera in"=w379) -> ("error out"=w374:errorcluster, "Interface.lvclass"=w375:refnum<class "Interface.lvclass">, "Simulated_CCD_Camera out"=w369:refnum<class "Simulated_CCD_Camera.lvclass">)  [unwired: 7 in]
              n175 = call "Read CCD Config.vi"("error in (no error)"=w374, "Interface in"=w375) -> ("error out"=w371:errorcluster, "Previous CCD Config"=w373:T1, "Interface out"=w370:refnum<class "Interface.lvclass">)  [unwired: 7 in]
              n176 = Bundle By Name(cluster=w373, "PREAMP"=w367) -> (w372:T1)
              n177 = call "Write CCD Config.vi"("error in (no error)"=w371, "CCD Config"=w372, "Interface in"=w370) -> ("error out"=w376:errorcluster, "Interface out"=w377:refnum<class "Interface.lvclass">)  [unwired: 7 in]
              n178 = call "Write Interface.lvclass.vi"("error in (no error)"=w376, "Interface.lvclass"=w377, "Simulated_CCD_Camera in"=w369) -> ("error out"=w381:errorcluster, "Simulated_CCD_Camera out"=w380:refnum<class "Simulated_CCD_Camera.lvclass">)  [unwired: 7 in]
              n179 = Bundle By Name(cluster=w384, "Simulated_CCD_Camera.lvclass"=w380) -> (w383:refnum<class "Channel.lvclass">)
            }
            frame "READOUT_RATE" {
              n180 = call "Read Tx Value.vi"("error in (no error)"=w406, "RxTx in"=w405) -> ("error out"=w398:errorcluster, "Rx Value"=w388:string)  [unwired: 7 in, 1 out]
              n181 = Unbundle By Name(w404) -> ("Simulated_CCD_Camera.lvclass"=w399:refnum<class "Simulated_CCD_Camera.lvclass">)
              n182 = Decimal String To Number(string=w388) -> (number=w387:i32)  [unwired: 2 in, 1 out]
              n183 = call "Read Interface.lvclass.vi"("error in (no error)"=w398, "Simulated_CCD_Camera in"=w399) -> ("error out"=w394:errorcluster, "Interface.lvclass"=w395:refnum<class "Interface.lvclass">, "Simulated_CCD_Camera out"=w389:refnum<class "Simulated_CCD_Camera.lvclass">)  [unwired: 7 in]
              n184 = call "Read CCD Config.vi"("error in (no error)"=w394, "Interface in"=w395) -> ("error out"=w391:errorcluster, "Previous CCD Config"=w393:T1, "Interface out"=w390:refnum<class "Interface.lvclass">)  [unwired: 7 in]
              n185 = Bundle By Name(cluster=w393, "READOUT_RATE"=w387) -> (w392:T1)
              n186 = call "Write CCD Config.vi"("error in (no error)"=w391, "CCD Config"=w392, "Interface in"=w390) -> ("error out"=w396:errorcluster, "Interface out"=w397:refnum<class "Interface.lvclass">)  [unwired: 7 in]
              n187 = call "Write Interface.lvclass.vi"("error in (no error)"=w396, "Interface.lvclass"=w397, "Simulated_CCD_Camera in"=w389) -> ("error out"=w401:errorcluster, "Simulated_CCD_Camera out"=w400:refnum<class "Simulated_CCD_Camera.lvclass">)  [unwired: 7 in]
              n188 = Bundle By Name(cluster=w404, "Simulated_CCD_Camera.lvclass"=w400) -> (w403:refnum<class "Channel.lvclass">)
            }
            frame "#FRAMES" {
              n189 = call "Read Tx Value.vi"("error in (no error)"=w426, "RxTx in"=w425) -> ("error out"=w418:errorcluster, "Rx Value"=w416:string)  [unwired: 7 in, 1 out]
              n190 = Unbundle By Name(w424) -> ("Simulated_CCD_Camera.lvclass"=w419:refnum<class "Simulated_CCD_Camera.lvclass">)
              n191 = Decimal String To Number(string=w416) -> (number=w407:i32)  [unwired: 2 in, 1 out]
              n192 = call "Read Interface.lvclass.vi"("error in (no error)"=w418, "Simulated_CCD_Camera in"=w419) -> ("error out"=w408:errorcluster, "Interface.lvclass"=w409:refnum<class "Interface.lvclass">, "Simulated_CCD_Camera out"=w417:refnum<class "Simulated_CCD_Camera.lvclass">)  [unwired: 7 in]
              n193 = call "Read SET parameters.vi"("error in (no error)"=w408, "Interface in"=w409) -> ("error out"=w411:errorcluster, "SET parameters"=w414:T8, "Interface out"=w410:refnum<class "Interface.lvclass">)  [unwired: 7 in]
              n194 = Bundle By Name(cluster=w414, "#FRAMES"=w407) -> (w415:T8)
              n195 = call "Write SET parameters.vi"("error in (no error)"=w411, "SET parameters"=w415, "Interface in"=w410) -> ("error out"=w412:errorcluster, "Interface out"=w413:refnum<class "Interface.lvclass">)  [unwired: 7 in]
              n196 = call "Write Interface.lvclass.vi"("error in (no error)"=w412, "Interface.lvclass"=w413, "Simulated_CCD_Camera in"=w417) -> ("error out"=w421:errorcluster, "Simulated_CCD_Camera out"=w420:refnum<class "Simulated_CCD_Camera.lvclass">)  [unwired: 7 in]
              n197 = Bundle By Name(cluster=w424, "Simulated_CCD_Camera.lvclass"=w420) -> (w423:refnum<class "Channel.lvclass">)
            }
            frame "#CUBES" {
              n198 = call "Read Tx Value.vi"("error in (no error)"=w446, "RxTx in"=w445) -> ("error out"=w438:errorcluster, "Rx Value"=w436:string)  [unwired: 7 in, 1 out]
              n199 = Unbundle By Name(w444) -> ("Simulated_CCD_Camera.lvclass"=w439:refnum<class "Simulated_CCD_Camera.lvclass">)
              n200 = Decimal String To Number(string=w436) -> (number=w427:i32)  [unwired: 2 in, 1 out]
              n201 = call "Read Interface.lvclass.vi"("error in (no error)"=w438, "Simulated_CCD_Camera in"=w439) -> ("error out"=w429:errorcluster, "Interface.lvclass"=w428:refnum<class "Interface.lvclass">, "Simulated_CCD_Camera out"=w437:refnum<class "Simulated_CCD_Camera.lvclass">)  [unwired: 7 in]
              n202 = call "Read SET parameters.vi"("error in (no error)"=w429, "Interface in"=w428) -> ("error out"=w430:errorcluster, "SET parameters"=w434:T8, "Interface out"=w431:refnum<class "Interface.lvclass">)  [unwired: 7 in]
              n203 = Bundle By Name(cluster=w434, "#CUBES"=w427) -> (w435:T8)
              n204 = call "Write SET parameters.vi"("error in (no error)"=w430, "SET parameters"=w435, "Interface in"=w431) -> ("error out"=w432:errorcluster, "Interface out"=w433:refnum<class "Interface.lvclass">)  [unwired: 7 in]
              n205 = call "Write Interface.lvclass.vi"("error in (no error)"=w432, "Interface.lvclass"=w433, "Simulated_CCD_Camera in"=w437) -> ("error out"=w441:errorcluster, "Simulated_CCD_Camera out"=w440:refnum<class "Simulated_CCD_Camera.lvclass">)  [unwired: 7 in]
              n206 = Bundle By Name(cluster=w444, "Simulated_CCD_Camera.lvclass"=w440) -> (w443:refnum<class "Channel.lvclass">)
            }
            frame "VBIN" {
              n207 = call "Read Tx Value.vi"("error in (no error)"=w466, "RxTx in"=w465) -> ("error out"=w458:errorcluster, "Rx Value"=w448:string)  [unwired: 7 in, 1 out]
              n208 = Unbundle By Name(w464) -> ("Simulated_CCD_Camera.lvclass"=w459:refnum<class "Simulated_CCD_Camera.lvclass">)
              n209 = Decimal String To Number(string=w448) -> (number=w447:i32)  [unwired: 2 in, 1 out]
              n210 = call "Read Interface.lvclass.vi"("error in (no error)"=w458, "Simulated_CCD_Camera in"=w459) -> ("error out"=w454:errorcluster, "Interface.lvclass"=w455:refnum<class "Interface.lvclass">, "Simulated_CCD_Camera out"=w449:refnum<class "Simulated_CCD_Camera.lvclass">)  [unwired: 7 in]
              n211 = call "Read CCD Config.vi"("error in (no error)"=w454, "Interface in"=w455) -> ("error out"=w451:errorcluster, "Previous CCD Config"=w453:T1, "Interface out"=w450:refnum<class "Interface.lvclass">)  [unwired: 7 in]
              n212 = Bundle By Name(cluster=w453, "VBIN"=w447) -> (w452:T1)
              n213 = call "Write CCD Config.vi"("error in (no error)"=w451, "CCD Config"=w452, "Interface in"=w450) -> ("error out"=w456:errorcluster, "Interface out"=w457:refnum<class "Interface.lvclass">)  [unwired: 7 in]
              n214 = call "Write Interface.lvclass.vi"("error in (no error)"=w456, "Interface.lvclass"=w457, "Simulated_CCD_Camera in"=w449) -> ("error out"=w461:errorcluster, "Simulated_CCD_Camera out"=w460:refnum<class "Simulated_CCD_Camera.lvclass">)  [unwired: 7 in]
              n215 = Bundle By Name(cluster=w464, "Simulated_CCD_Camera.lvclass"=w460) -> (w463:refnum<class "Channel.lvclass">)
            }
            frame "HBIN" {
              n216 = call "Read Tx Value.vi"("error in (no error)"=w486, "RxTx in"=w485) -> ("error out"=w478:errorcluster, "Rx Value"=w468:string)  [unwired: 7 in, 1 out]
              n217 = Unbundle By Name(w484) -> ("Simulated_CCD_Camera.lvclass"=w479:refnum<class "Simulated_CCD_Camera.lvclass">)
              n218 = Decimal String To Number(string=w468) -> (number=w467:i32)  [unwired: 2 in, 1 out]
              n219 = call "Read Interface.lvclass.vi"("error in (no error)"=w478, "Simulated_CCD_Camera in"=w479) -> ("error out"=w474:errorcluster, "Interface.lvclass"=w475:refnum<class "Interface.lvclass">, "Simulated_CCD_Camera out"=w469:refnum<class "Simulated_CCD_Camera.lvclass">)  [unwired: 7 in]
              n220 = call "Read CCD Config.vi"("error in (no error)"=w474, "Interface in"=w475) -> ("error out"=w471:errorcluster, "Previous CCD Config"=w473:T1, "Interface out"=w470:refnum<class "Interface.lvclass">)  [unwired: 7 in]
              n221 = Bundle By Name(cluster=w473, "HBIN"=w467) -> (w472:T1)
              n222 = call "Write CCD Config.vi"("error in (no error)"=w471, "CCD Config"=w472, "Interface in"=w470) -> ("error out"=w476:errorcluster, "Interface out"=w477:refnum<class "Interface.lvclass">)  [unwired: 7 in]
              n223 = call "Write Interface.lvclass.vi"("error in (no error)"=w476, "Interface.lvclass"=w477, "Simulated_CCD_Camera in"=w469) -> ("error out"=w481:errorcluster, "Simulated_CCD_Camera out"=w480:refnum<class "Simulated_CCD_Camera.lvclass">)  [unwired: 7 in]
              n224 = Bundle By Name(cluster=w484, "Simulated_CCD_Camera.lvclass"=w480) -> (w483:refnum<class "Channel.lvclass">)
            }
            frame "EM_GAIN" {
              n225 = call "Read Tx Value.vi"("error in (no error)"=w506, "RxTx in"=w505) -> ("error out"=w498:errorcluster, "Rx Value"=w488:string)  [unwired: 7 in, 1 out]
              n226 = Unbundle By Name(w504) -> ("Simulated_CCD_Camera.lvclass"=w499:refnum<class "Simulated_CCD_Camera.lvclass">)
              n227 = Decimal String To Number(string=w488) -> (number=w487:i32)  [unwired: 2 in, 1 out]
              n228 = call "Read Interface.lvclass.vi"("error in (no error)"=w498, "Simulated_CCD_Camera in"=w499) -> ("error out"=w494:errorcluster, "Interface.lvclass"=w495:refnum<class "Interface.lvclass">, "Simulated_CCD_Camera out"=w489:refnum<class "Simulated_CCD_Camera.lvclass">)  [unwired: 7 in]
              n229 = call "Read CCD Config.vi"("error in (no error)"=w494, "Interface in"=w495) -> ("error out"=w491:errorcluster, "Previous CCD Config"=w493:T1, "Interface out"=w490:refnum<class "Interface.lvclass">)  [unwired: 7 in]
              n230 = Bundle By Name(cluster=w493, "EM_GAIN"=w487) -> (w492:T1)
              n231 = call "Write CCD Config.vi"("error in (no error)"=w491, "CCD Config"=w492, "Interface in"=w490) -> ("error out"=w496:errorcluster, "Interface out"=w497:refnum<class "Interface.lvclass">)  [unwired: 7 in]
              n232 = call "Write Interface.lvclass.vi"("error in (no error)"=w496, "Interface.lvclass"=w497, "Simulated_CCD_Camera in"=w489) -> ("error out"=w501:errorcluster, "Simulated_CCD_Camera out"=w500:refnum<class "Simulated_CCD_Camera.lvclass">)  [unwired: 7 in]
              n233 = Bundle By Name(cluster=w504, "Simulated_CCD_Camera.lvclass"=w500) -> (w503:refnum<class "Channel.lvclass">)
            }
            frame "EM_MODE" {
              n234 = call "Read Tx Value.vi"("error in (no error)"=w526, "RxTx in"=w525) -> ("error out"=w518:errorcluster, "Rx Value"=w508:string)  [unwired: 7 in, 1 out]
              n235 = Unbundle By Name(w524) -> ("Simulated_CCD_Camera.lvclass"=w519:refnum<class "Simulated_CCD_Camera.lvclass">)
              n236 = Decimal String To Number(string=w508) -> (number=w507:i32)  [unwired: 2 in, 1 out]
              n237 = call "Read Interface.lvclass.vi"("error in (no error)"=w518, "Simulated_CCD_Camera in"=w519) -> ("error out"=w514:errorcluster, "Interface.lvclass"=w515:refnum<class "Interface.lvclass">, "Simulated_CCD_Camera out"=w509:refnum<class "Simulated_CCD_Camera.lvclass">)  [unwired: 7 in]
              n238 = call "Read CCD Config.vi"("error in (no error)"=w514, "Interface in"=w515) -> ("error out"=w511:errorcluster, "Previous CCD Config"=w513:T1, "Interface out"=w510:refnum<class "Interface.lvclass">)  [unwired: 7 in]
              n239 = Bundle By Name(cluster=w513, "EM_MODE"=w507) -> (w512:T1)
              n240 = call "Write CCD Config.vi"("error in (no error)"=w511, "CCD Config"=w512, "Interface in"=w510) -> ("error out"=w516:errorcluster, "Interface out"=w517:refnum<class "Interface.lvclass">)  [unwired: 7 in]
              n241 = call "Write Interface.lvclass.vi"("error in (no error)"=w516, "Interface.lvclass"=w517, "Simulated_CCD_Camera in"=w509) -> ("error out"=w521:errorcluster, "Simulated_CCD_Camera out"=w520:refnum<class "Simulated_CCD_Camera.lvclass">)  [unwired: 7 in]
              n242 = Bundle By Name(cluster=w524, "Simulated_CCD_Camera.lvclass"=w520) -> (w523:refnum<class "Channel.lvclass">)
            }
            frame "FINAL_COLUMN" {
              n243 = call "Read Tx Value.vi"("error in (no error)"=w546, "RxTx in"=w545) -> ("error out"=w538:errorcluster, "Rx Value"=w528:string)  [unwired: 7 in, 1 out]
              n244 = Unbundle By Name(w544) -> ("Simulated_CCD_Camera.lvclass"=w539:refnum<class "Simulated_CCD_Camera.lvclass">)
              n245 = Decimal String To Number(string=w528) -> (number=w527:i32)  [unwired: 2 in, 1 out]
              n246 = call "Read Interface.lvclass.vi"("error in (no error)"=w538, "Simulated_CCD_Camera in"=w539) -> ("error out"=w534:errorcluster, "Interface.lvclass"=w535:refnum<class "Interface.lvclass">, "Simulated_CCD_Camera out"=w529:refnum<class "Simulated_CCD_Camera.lvclass">)  [unwired: 7 in]
              n247 = call "Read CCD Config.vi"("error in (no error)"=w534, "Interface in"=w535) -> ("error out"=w531:errorcluster, "Previous CCD Config"=w533:T1, "Interface out"=w530:refnum<class "Interface.lvclass">)  [unwired: 7 in]
              n248 = Bundle By Name(cluster=w533, "FINAL_COLUMN"=w527) -> (w532:T1)
              n249 = call "Write CCD Config.vi"("error in (no error)"=w531, "CCD Config"=w532, "Interface in"=w530) -> ("error out"=w536:errorcluster, "Interface out"=w537:refnum<class "Interface.lvclass">)  [unwired: 7 in]
              n250 = call "Write Interface.lvclass.vi"("error in (no error)"=w536, "Interface.lvclass"=w537, "Simulated_CCD_Camera in"=w529) -> ("error out"=w541:errorcluster, "Simulated_CCD_Camera out"=w540:refnum<class "Simulated_CCD_Camera.lvclass">)  [unwired: 7 in]
              n251 = Bundle By Name(cluster=w544, "Simulated_CCD_Camera.lvclass"=w540) -> (w543:refnum<class "Channel.lvclass">)
            }
            frame "FINAL_LINE" {
              n252 = call "Read Tx Value.vi"("error in (no error)"=w566, "RxTx in"=w565) -> ("error out"=w558:errorcluster, "Rx Value"=w548:string)  [unwired: 7 in, 1 out]
              n253 = Unbundle By Name(w564) -> ("Simulated_CCD_Camera.lvclass"=w559:refnum<class "Simulated_CCD_Camera.lvclass">)
              n254 = Decimal String To Number(string=w548) -> (number=w547:i32)  [unwired: 2 in, 1 out]
              n255 = call "Read Interface.lvclass.vi"("error in (no error)"=w558, "Simulated_CCD_Camera in"=w559) -> ("error out"=w554:errorcluster, "Interface.lvclass"=w555:refnum<class "Interface.lvclass">, "Simulated_CCD_Camera out"=w549:refnum<class "Simulated_CCD_Camera.lvclass">)  [unwired: 7 in]
              n256 = call "Read CCD Config.vi"("error in (no error)"=w554, "Interface in"=w555) -> ("error out"=w551:errorcluster, "Previous CCD Config"=w553:T1, "Interface out"=w550:refnum<class "Interface.lvclass">)  [unwired: 7 in]
              n257 = Bundle By Name(cluster=w553, "FINAL_LINE"=w547) -> (w552:T1)
              n258 = call "Write CCD Config.vi"("error in (no error)"=w551, "CCD Config"=w552, "Interface in"=w550) -> ("error out"=w556:errorcluster, "Interface out"=w557:refnum<class "Interface.lvclass">)  [unwired: 7 in]
              n259 = call "Write Interface.lvclass.vi"("error in (no error)"=w556, "Interface.lvclass"=w557, "Simulated_CCD_Camera in"=w549) -> ("error out"=w561:errorcluster, "Simulated_CCD_Camera out"=w560:refnum<class "Simulated_CCD_Camera.lvclass">)  [unwired: 7 in]
              n260 = Bundle By Name(cluster=w564, "Simulated_CCD_Camera.lvclass"=w560) -> (w563:refnum<class "Channel.lvclass">)
            }
            frame "INITIAL_COLUMN" {
              n261 = call "Read Tx Value.vi"("error in (no error)"=w586, "RxTx in"=w585) -> ("error out"=w578:errorcluster, "Rx Value"=w568:string)  [unwired: 7 in, 1 out]
              n262 = Unbundle By Name(w584) -> ("Simulated_CCD_Camera.lvclass"=w579:refnum<class "Simulated_CCD_Camera.lvclass">)
              n263 = Decimal String To Number(string=w568) -> (number=w567:i32)  [unwired: 2 in, 1 out]
              n264 = call "Read Interface.lvclass.vi"("error in (no error)"=w578, "Simulated_CCD_Camera in"=w579) -> ("error out"=w574:errorcluster, "Interface.lvclass"=w575:refnum<class "Interface.lvclass">, "Simulated_CCD_Camera out"=w569:refnum<class "Simulated_CCD_Camera.lvclass">)  [unwired: 7 in]
              n265 = call "Read CCD Config.vi"("error in (no error)"=w574, "Interface in"=w575) -> ("error out"=w571:errorcluster, "Previous CCD Config"=w573:T1, "Interface out"=w570:refnum<class "Interface.lvclass">)  [unwired: 7 in]
              n266 = Bundle By Name(cluster=w573, "INITIAL_COLUMN"=w567) -> (w572:T1)
              n267 = call "Write CCD Config.vi"("error in (no error)"=w571, "CCD Config"=w572, "Interface in"=w570) -> ("error out"=w576:errorcluster, "Interface out"=w577:refnum<class "Interface.lvclass">)  [unwired: 7 in]
              n268 = call "Write Interface.lvclass.vi"("error in (no error)"=w576, "Interface.lvclass"=w577, "Simulated_CCD_Camera in"=w569) -> ("error out"=w581:errorcluster, "Simulated_CCD_Camera out"=w580:refnum<class "Simulated_CCD_Camera.lvclass">)  [unwired: 7 in]
              n269 = Bundle By Name(cluster=w584, "Simulated_CCD_Camera.lvclass"=w580) -> (w583:refnum<class "Channel.lvclass">)
            }
            frame "INITIAL_LINE" {
              n270 = call "Read Tx Value.vi"("error in (no error)"=w606, "RxTx in"=w605) -> ("error out"=w598:errorcluster, "Rx Value"=w588:string)  [unwired: 7 in, 1 out]
              n271 = Unbundle By Name(w604) -> ("Simulated_CCD_Camera.lvclass"=w599:refnum<class "Simulated_CCD_Camera.lvclass">)
              n272 = Decimal String To Number(string=w588) -> (number=w587:i32)  [unwired: 2 in, 1 out]
              n273 = call "Read Interface.lvclass.vi"("error in (no error)"=w598, "Simulated_CCD_Camera in"=w599) -> ("error out"=w594:errorcluster, "Interface.lvclass"=w595:refnum<class "Interface.lvclass">, "Simulated_CCD_Camera out"=w589:refnum<class "Simulated_CCD_Camera.lvclass">)  [unwired: 7 in]
              n274 = call "Read CCD Config.vi"("error in (no error)"=w594, "Interface in"=w595) -> ("error out"=w591:errorcluster, "Previous CCD Config"=w593:T1, "Interface out"=w590:refnum<class "Interface.lvclass">)  [unwired: 7 in]
              n275 = Bundle By Name(cluster=w593, "INITIAL_LINE"=w587) -> (w592:T1)
              n276 = call "Write CCD Config.vi"("error in (no error)"=w591, "CCD Config"=w592, "Interface in"=w590) -> ("error out"=w596:errorcluster, "Interface out"=w597:refnum<class "Interface.lvclass">)  [unwired: 7 in]
              n277 = call "Write Interface.lvclass.vi"("error in (no error)"=w596, "Interface.lvclass"=w597, "Simulated_CCD_Camera in"=w589) -> ("error out"=w601:errorcluster, "Simulated_CCD_Camera out"=w600:refnum<class "Simulated_CCD_Camera.lvclass">)  [unwired: 7 in]
              n278 = Bundle By Name(cluster=w604, "Simulated_CCD_Camera.lvclass"=w600) -> (w603:refnum<class "Channel.lvclass">)
            }
            frame "TRIGGER_MODE" {
              n279 = call "Read Tx Value.vi"("error in (no error)"=w626, "RxTx in"=w625) -> ("error out"=w618:errorcluster, "Rx Value"=w608:string)  [unwired: 7 in, 1 out]
              n280 = Unbundle By Name(w624) -> ("Simulated_CCD_Camera.lvclass"=w619:refnum<class "Simulated_CCD_Camera.lvclass">)
              n281 = Decimal String To Number(string=w608) -> (number=w607:i32)  [unwired: 2 in, 1 out]
              n282 = call "Read Interface.lvclass.vi"("error in (no error)"=w618, "Simulated_CCD_Camera in"=w619) -> ("error out"=w614:errorcluster, "Interface.lvclass"=w615:refnum<class "Interface.lvclass">, "Simulated_CCD_Camera out"=w609:refnum<class "Simulated_CCD_Camera.lvclass">)  [unwired: 7 in]
              n283 = call "Read CCD Config.vi"("error in (no error)"=w614, "Interface in"=w615) -> ("error out"=w611:errorcluster, "Previous CCD Config"=w613:T1, "Interface out"=w610:refnum<class "Interface.lvclass">)  [unwired: 7 in]
              n284 = Bundle By Name(cluster=w613, "TRIGGER_MODE"=w607) -> (w612:T1)
              n285 = call "Write CCD Config.vi"("error in (no error)"=w611, "CCD Config"=w612, "Interface in"=w610) -> ("error out"=w616:errorcluster, "Interface out"=w617:refnum<class "Interface.lvclass">)  [unwired: 7 in]
              n286 = call "Write Interface.lvclass.vi"("error in (no error)"=w616, "Interface.lvclass"=w617, "Simulated_CCD_Camera in"=w609) -> ("error out"=w621:errorcluster, "Simulated_CCD_Camera out"=w620:refnum<class "Simulated_CCD_Camera.lvclass">)  [unwired: 7 in]
              n287 = Bundle By Name(cluster=w624, "Simulated_CCD_Camera.lvclass"=w620) -> (w623:refnum<class "Channel.lvclass">)
            }
            frame "SHUTTER_MODE" {
              n288 = call "Read Tx Value.vi"("error in (no error)"=w646, "RxTx in"=w645) -> ("error out"=w638:errorcluster, "Rx Value"=w628:string)  [unwired: 7 in, 1 out]
              n289 = Unbundle By Name(w644) -> ("Simulated_CCD_Camera.lvclass"=w639:refnum<class "Simulated_CCD_Camera.lvclass">)
              n290 = Decimal String To Number(string=w628) -> (number=w627:i32)  [unwired: 2 in, 1 out]
              n291 = call "Read Interface.lvclass.vi"("error in (no error)"=w638, "Simulated_CCD_Camera in"=w639) -> ("error out"=w634:errorcluster, "Interface.lvclass"=w635:refnum<class "Interface.lvclass">, "Simulated_CCD_Camera out"=w629:refnum<class "Simulated_CCD_Camera.lvclass">)  [unwired: 7 in]
              n292 = call "Read CCD Config.vi"("error in (no error)"=w634, "Interface in"=w635) -> ("error out"=w631:errorcluster, "Previous CCD Config"=w633:T1, "Interface out"=w630:refnum<class "Interface.lvclass">)  [unwired: 7 in]
              n293 = Bundle By Name(cluster=w633, "SHUTTER_MODE"=w627) -> (w632:T1)
              n294 = call "Write CCD Config.vi"("error in (no error)"=w631, "CCD Config"=w632, "Interface in"=w630) -> ("error out"=w636:errorcluster, "Interface out"=w637:refnum<class "Interface.lvclass">)  [unwired: 7 in]
              n295 = call "Write Interface.lvclass.vi"("error in (no error)"=w636, "Interface.lvclass"=w637, "Simulated_CCD_Camera in"=w629) -> ("error out"=w641:errorcluster, "Simulated_CCD_Camera out"=w640:refnum<class "Simulated_CCD_Camera.lvclass">)  [unwired: 7 in]
              n296 = Bundle By Name(cluster=w644, "Simulated_CCD_Camera.lvclass"=w640) -> (w643:refnum<class "Channel.lvclass">)
            }
            frame "TEMP" {
              n297 = call "Read Tx Value.vi"("error in (no error)"=w666, "RxTx in"=w665) -> ("error out"=w656:errorcluster, "Rx Value"=w664:string)  [unwired: 7 in, 1 out]
              n298 = Unbundle By Name(w667) -> ("Simulated_CCD_Camera.lvclass"=w657:refnum<class "Simulated_CCD_Camera.lvclass">)
              n299 = call "Read Interface.lvclass.vi"("error in (no error)"=w656, "Simulated_CCD_Camera in"=w657) -> ("error out"=w652:errorcluster, "Interface.lvclass"=w653:refnum<class "Interface.lvclass">, "Simulated_CCD_Camera out"=w662:refnum<class "Simulated_CCD_Camera.lvclass">)  [unwired: 7 in]
              n300 = Decimal String To Number(string=w664) -> (number=w647:i32)  [unwired: 2 in, 1 out]
              n301 = call "Read SET parameters.vi"("error in (no error)"=w652, "Interface in"=w653) -> ("error out"=w648:errorcluster, "SET parameters"=w655:T8, "Interface out"=w649:refnum<class "Interface.lvclass">)  [unwired: 7 in]
              n302 = Bundle By Name(cluster=w655, "TEMP"=w647) -> (w654:T8)
              n303 = call "Write SET parameters.vi"("error in (no error)"=w648, "SET parameters"=w654, "Interface in"=w649) -> ("error out"=w651:errorcluster, "Interface out"=w650:refnum<class "Interface.lvclass">)  [unwired: 7 in]
              n304 = call "Write Interface.lvclass.vi"("error in (no error)"=w651, "Interface.lvclass"=w650, "Simulated_CCD_Camera in"=w662) -> ("error out"=w660:errorcluster, "Simulated_CCD_Camera out"=w661:refnum<class "Simulated_CCD_Camera.lvclass">)  [unwired: 7 in]
              n305 = call-dynamic "Set Temperature.vi"("error in (no error)"=w660, "Simulated_CCD_Camera in"=w661) -> ("error out"=w658:errorcluster, "Simulated_CCD_Camera out"=w659:refnum<class "Simulated_CCD_Camera.lvclass">)  [unwired: 8 in]
              n306 = Bundle By Name(cluster=w667, "Simulated_CCD_Camera.lvclass"=w659) -> (w668:refnum<class "Channel.lvclass">)
            }
            frame "COMMENT" {
              n307 = call "Read Tx Value.vi"("error in (no error)"=w679, "RxTx in"=w680) -> ("error out"=w670:errorcluster, "Rx Value"=w669:string)  [unwired: 7 in, 1 out]
              n308 = Unbundle By Name(w681) -> ("Save Image.lvclass"=w673:refnum<class "Save Image.lvclass">)
              n309 = call "Read Header parameters.vi"("error in (no error)"=w670, "Save Image in"=w673) -> ("error out"=w677:errorcluster, "Header parameters"=w674:T7, "Save Image out"=w676:refnum<class "Save Image.lvclass">)  [unwired: 7 in]
              n310 = Bundle By Name(cluster=w674, "COMNENT"=w669) -> (w675:T7)
              n311 = call "Write Header parameters.vi"("error in (no error)"=w677, "Header parameters"=w675, "Save Image in"=w676) -> ("error out"=w671:errorcluster, "Save Image out"=w672:refnum<class "Save Image.lvclass">)  [unwired: 7 in]
              n312 = Bundle By Name(cluster=w681, "Save Image.lvclass"=w672) -> (w682:refnum<class "Channel.lvclass">)
            }
            frame "SUFFIX" {
              n313 = call "Read Tx Value.vi"("error in (no error)"=w689, "RxTx in"=w690) -> ("error out"=w684:errorcluster, "Rx Value"=w688:string)  [unwired: 7 in, 1 out]
              n314 = Unbundle By Name(w691) -> ("Save Image.lvclass"=w685:refnum<class "Save Image.lvclass">)
              n315 = call "Write Suffix image name.vi"("error in (no error)"=w684, "Suffix image name"=w688, "Save Image in"=w685) -> ("error out"=w683:errorcluster, "Save Image out"=w686:refnum<class "Save Image.lvclass">)  [unwired: 7 in]
              n316 = Bundle By Name(cluster=w691, "Save Image.lvclass"=w686) -> (w692:refnum<class "Channel.lvclass">)
            }
            frame "OBSTYPE" {
              n317 = call "Read Tx Value.vi"("error in (no error)"=w703, "RxTx in"=w704) -> ("error out"=w694:errorcluster, "Rx Value"=w693:string)  [unwired: 7 in, 1 out]
              n318 = Unbundle By Name(w705) -> ("Save Image.lvclass"=w697:refnum<class "Save Image.lvclass">)
              n319 = call "Read Header parameters.vi"("error in (no error)"=w694, "Save Image in"=w697) -> ("error out"=w700:errorcluster, "Header parameters"=w698:T7, "Save Image out"=w701:refnum<class "Save Image.lvclass">)  [unwired: 7 in]
              n320 = Bundle By Name(cluster=w698, "OBSTYPE"=w693) -> (w699:T7)
              n321 = call "Write Header parameters.vi"("error in (no error)"=w700, "Header parameters"=w699, "Save Image in"=w701) -> ("error out"=w695:errorcluster, "Save Image out"=w696:refnum<class "Save Image.lvclass">)  [unwired: 7 in]
              n322 = Bundle By Name(cluster=w705, "Save Image.lvclass"=w696) -> (w706:refnum<class "Channel.lvclass">)
            }
            frame "COOLER_POWER_STATUS" {
              n323 = call "Read Tx Value.vi"("error in (no error)"=w726, "RxTx in"=w725) -> ("error out"=w716:errorcluster, "Rx Value"=w723:string)  [unwired: 7 in, 1 out]
              n324 = Unbundle By Name(w727) -> ("Simulated_CCD_Camera.lvclass"=w717:refnum<class "Simulated_CCD_Camera.lvclass">)
              n325 = Decimal String To Number(string=w723) -> (number=w707:i32)  [unwired: 2 in, 1 out]
              n326 = call "Read Interface.lvclass.vi"("error in (no error)"=w716, "Simulated_CCD_Camera in"=w717) -> ("error out"=w708:errorcluster, "Interface.lvclass"=w709:refnum<class "Interface.lvclass">, "Simulated_CCD_Camera out"=w722:refnum<class "Simulated_CCD_Camera.lvclass">)  [unwired: 7 in]
              n327 = call "Read SET parameters.vi"("error in (no error)"=w708, "Interface in"=w709) -> ("error out"=w711:errorcluster, "SET parameters"=w715:T8, "Interface out"=w710:refnum<class "Interface.lvclass">)  [unwired: 7 in]
              n328 = Bundle By Name(cluster=w715, "COOLER_POWER_STATUS"=w707) -> (w714:T8)
              n329 = call "Write SET parameters.vi"("error in (no error)"=w711, "SET parameters"=w714, "Interface in"=w710) -> ("error out"=w712:errorcluster, "Interface out"=w713:refnum<class "Interface.lvclass">)  [unwired: 7 in]
              n330 = call "Write Interface.lvclass.vi"("error in (no error)"=w712, "Interface.lvclass"=w713, "Simulated_CCD_Camera in"=w722) -> ("error out"=w720:errorcluster, "Simulated_CCD_Camera out"=w721:refnum<class "Simulated_CCD_Camera.lvclass">)  [unwired: 7 in]
              n331 = call-dynamic "Set Cooler Power Status.vi"("error in (no error)"=w720, "Simulated_CCD_Camera in"=w721) -> ("error out"=w718:errorcluster, "Simulated_CCD_Camera out"=w719:refnum<class "Simulated_CCD_Camera.lvclass">)  [unwired: 8 in]
              n332 = Bundle By Name(cluster=w727, "Simulated_CCD_Camera.lvclass"=w719) -> (w728:refnum<class "Channel.lvclass">)
            }
          }
          n333 = Unbundle By Name(w327) -> ("Simulated_CCD_Camera.lvclass"=w328:refnum<class "Simulated_CCD_Camera.lvclass">)
          n334 = call-dynamic "Set Camera Configuration.vi"("error in (no error)"=w323, "CCDCamera in"=w328) -> ("error out"=w324:errorcluster, "CCDCamera out"=w326:refnum<class "Simulated_CCD_Camera.lvclass">)  [unwired: 8 in]
          n335 = Bundle By Name(cluster=w327, "Simulated_CCD_Camera.lvclass"=w326) -> (w325:refnum<class "Channel.lvclass">)
          n336 = Unbundle By Name(w325) -> ("RxTx.lvclass"=w338:refnum<class "RxTx.lvclass">)
          n337 = call "Send TX Message.vi"("error in (no error)"=w324, "element"=w336, "RxTx in"=w338) -> ("error out"=w330:errorcluster, "RxTx out"=w337:refnum<class "RxTx.lvclass">)  [unwired: 7 in]
          n338 = Bundle By Name(cluster=w325, "RxTx.lvclass"=w337) -> (w329:refnum<class "Channel.lvclass">)
          n339 = Unbundle By Name(w329) -> ("State Machine.lvclass"=w332:refnum<class "State Machine.lvclass">)
          n340 = call-dynamic "Write State.vi"("error in (no error)"=w330, "State"="False", "State Machine in"=w332) -> ("error out"=w321:errorcluster, "State Machine out"=w333:refnum<class "State Machine.lvclass">)  [unwired: 7 in]
          n341 = Bundle By Name(cluster=w329, "State Machine.lvclass"=w333) -> (w322:refnum<class "Channel.lvclass">)
        }
        frame "GET" {
          n342 = Unbundle By Name(w738) -> ("RxTx.lvclass"=w744:refnum<class "RxTx.lvclass">)
          n343 = call "Read Rx Value.vi"("error in (no error)"=w737, "RxTx in"=w744) -> ("error out"=w745:errorcluster, "Rx value"=w729:string)  [unwired: 7 in, 1 out]
          n344 = case shown="\"#FRAMES\"" w729 {
            tunnel: [w748 w757 w766 w775 w784 w793 w802 w811 w820 w829 w838 w847 w853 w858 w864 w873 w882 w891 w900 w909] -> w741
            tunnel: w738 -> [w748 w757 w766 w775 w784 w793 w802 w811 w820 w829 w838 w847 w853 w858 w864 w873 w882 w891 w900 w909]
            tunnel: [w747 w749 w758 w767 w776 w785 w794 w803 w812 w821 w830 w839 w849 w857 w860 w866 w875 w884 w893 w901] -> w740
            tunnel: w745 -> [w747 w754 w763 w772 w781 w790 w799 w808 w817 w826 w835 w844 w850 w855 w859 w867 w876 w885 w897 w906]
            tunnel: ["INVALID_PARAMETER" w756 w765 w774 w783 w792 w801 w810 w819 w828 w837 w846 w848 w856 w861 w872 w881 w890 w899 w908] -> w739
            frame "False", Default {
            }
            frame "EXPTIME" {
              n345 = Unbundle By Name(w757) -> ("Simulated_CCD_Camera.lvclass"=w755:refnum<class "Simulated_CCD_Camera.lvclass">)
              n346 = call "Read Interface.lvclass.vi"("error in (no error)"=w754, "Simulated_CCD_Camera in"=w755) -> ("error out"=w752:errorcluster, "Interface.lvclass"=w753:refnum<class "Interface.lvclass">)  [unwired: 7 in, 1 out]
              n347 = call "Read Previous SET parameters.vi"("error in (no error)"=w752, "Interface in"=w753) -> ("error out"=w749:errorcluster, "Previous SET parameters"=w751:T8)  [unwired: 7 in, 1 out]
              n348 = Unbundle By Name(w751) -> ("EXPTIME"=w750:dbl)
              n349 = Number To Fractional String(number=w750) -> (F-format string=w756:string)  [unwired: 3 in]
            }
            frame "READOUT_RATE" {
              n350 = Unbundle By Name(w766) -> ("Simulated_CCD_Camera.lvclass"=w764:refnum<class "Simulated_CCD_Camera.lvclass">)
              n351 = call "Read Interface.lvclass.vi"("error in (no error)"=w763, "Simulated_CCD_Camera in"=w764) -> ("error out"=w761:errorcluster, "Interface.lvclass"=w762:refnum<class "Interface.lvclass">)  [unwired: 7 in, 1 out]
              n352 = call "Read Previous CCD Config.vi"("error in (no error)"=w761, "Interface in"=w762) -> ("error out"=w758:errorcluster, "Previous CCD Config"=w760:T6)  [unwired: 7 in, 1 out]
              n353 = Unbundle By Name(w760) -> ("READOUT_RATE"=w759:enum16{"30 MHz", "20 MHz", "10 MHz", "1 MHz"})
              n354 = Number To Fractional String(number=w759) -> (F-format string=w765:string)  [unwired: 3 in]
            }
            frame "VBIN" {
              n355 = Unbundle By Name(w775) -> ("Simulated_CCD_Camera.lvclass"=w773:refnum<class "Simulated_CCD_Camera.lvclass">)
              n356 = call "Read Interface.lvclass.vi"("error in (no error)"=w772, "Simulated_CCD_Camera in"=w773) -> ("error out"=w770:errorcluster, "Interface.lvclass"=w771:refnum<class "Interface.lvclass">)  [unwired: 7 in, 1 out]
              n357 = call "Read Previous CCD Config.vi"("error in (no error)"=w770, "Interface in"=w771) -> ("error out"=w767:errorcluster, "Previous CCD Config"=w769:T6)  [unwired: 7 in, 1 out]
              n358 = Unbundle By Name(w769) -> ("VBIN"=w768:u16)
              n359 = Number To Fractional String(number=w768) -> (F-format string=w774:string)  [unwired: 3 in]
            }
            frame "HBIN" {
              n360 = Unbundle By Name(w784) -> ("Simulated_CCD_Camera.lvclass"=w782:refnum<class "Simulated_CCD_Camera.lvclass">)
              n361 = call "Read Interface.lvclass.vi"("error in (no error)"=w781, "Simulated_CCD_Camera in"=w782) -> ("error out"=w779:errorcluster, "Interface.lvclass"=w780:refnum<class "Interface.lvclass">)  [unwired: 7 in, 1 out]
              n362 = call "Read Previous CCD Config.vi"("error in (no error)"=w779, "Interface in"=w780) -> ("error out"=w776:errorcluster, "Previous CCD Config"=w778:T6)  [unwired: 7 in, 1 out]
              n363 = Unbundle By Name(w778) -> ("HBIN"=w777:u16)
              n364 = Number To Fractional String(number=w777) -> (F-format string=w783:string)  [unwired: 3 in]
            }
            frame "COOLER_POWER_STATUS" {
              n365 = Unbundle By Name(w793) -> ("Simulated_CCD_Camera.lvclass"=w791:refnum<class "Simulated_CCD_Camera.lvclass">)
              n366 = call "Read Interface.lvclass.vi"("error in (no error)"=w790, "Simulated_CCD_Camera in"=w791) -> ("error out"=w788:errorcluster, "Interface.lvclass"=w789:refnum<class "Interface.lvclass">)  [unwired: 7 in, 1 out]
              n367 = call "Read Previous SET parameters.vi"("error in (no error)"=w788, "Interface in"=w789) -> ("error out"=w785:errorcluster, "Previous SET parameters"=w787:T8)  [unwired: 7 in, 1 out]
              n368 = Unbundle By Name(w787) -> ("COOLER_POWER_STATUS"=w786:u16)
              n369 = Number To Fractional String(number=w786) -> (F-format string=w792:string)  [unwired: 3 in]
            }
            frame "EM_GAIN" {
              n370 = Unbundle By Name(w802) -> ("Simulated_CCD_Camera.lvclass"=w800:refnum<class "Simulated_CCD_Camera.lvclass">)
              n371 = call "Read Interface.lvclass.vi"("error in (no error)"=w799, "Simulated_CCD_Camera in"=w800) -> ("error out"=w797:errorcluster, "Interface.lvclass"=w798:refnum<class "Interface.lvclass">)  [unwired: 7 in, 1 out]
              n372 = call "Read Previous CCD Config.vi"("error in (no error)"=w797, "Interface in"=w798) -> ("error out"=w794:errorcluster, "Previous CCD Config"=w796:T6)  [unwired: 7 in, 1 out]
              n373 = Unbundle By Name(w796) -> ("EM_GAIN"=w795:u16)
              n374 = Number To Fractional String(number=w795) -> (F-format string=w801:string)  [unwired: 3 in]
            }
            frame "EM_MODE" {
              n375 = Unbundle By Name(w811) -> ("Simulated_CCD_Camera.lvclass"=w809:refnum<class "Simulated_CCD_Camera.lvclass">)
              n376 = call "Read Interface.lvclass.vi"("error in (no error)"=w808, "Simulated_CCD_Camera in"=w809) -> ("error out"=w806:errorcluster, "Interface.lvclass"=w807:refnum<class "Interface.lvclass">)  [unwired: 7 in, 1 out]
              n377 = call "Read Previous CCD Config.vi"("error in (no error)"=w806, "Interface in"=w807) -> ("error out"=w803:errorcluster, "Previous CCD Config"=w805:T6)  [unwired: 7 in, 1 out]
              n378 = Unbundle By Name(w805) -> ("EM_MODE"=w804:enum16{"Electron Multiplying", "Conventional"})
              n379 = Number To Fractional String(number=w804) -> (F-format string=w810:string)  [unwired: 3 in]
            }
            frame "FINAL_COLUMN" {
              n380 = Unbundle By Name(w820) -> ("Simulated_CCD_Camera.lvclass"=w818:refnum<class "Simulated_CCD_Camera.lvclass">)
              n381 = call "Read Interface.lvclass.vi"("error in (no error)"=w817, "Simulated_CCD_Camera in"=w818) -> ("error out"=w815:errorcluster, "Interface.lvclass"=w816:refnum<class "Interface.lvclass">)  [unwired: 7 in, 1 out]
              n382 = call "Read Previous CCD Config.vi"("error in (no error)"=w815, "Interface in"=w816) -> ("error out"=w812:errorcluster, "Previous CCD Config"=w814:T6)  [unwired: 7 in, 1 out]
              n383 = Unbundle By Name(w814) -> ("FINAL_COLUMN"=w813:u16)
              n384 = Number To Fractional String(number=w813) -> (F-format string=w819:string)  [unwired: 3 in]
            }
            frame "FINAL_LINE" {
              n385 = Unbundle By Name(w829) -> ("Simulated_CCD_Camera.lvclass"=w827:refnum<class "Simulated_CCD_Camera.lvclass">)
              n386 = call "Read Interface.lvclass.vi"("error in (no error)"=w826, "Simulated_CCD_Camera in"=w827) -> ("error out"=w824:errorcluster, "Interface.lvclass"=w825:refnum<class "Interface.lvclass">)  [unwired: 7 in, 1 out]
              n387 = call "Read Previous CCD Config.vi"("error in (no error)"=w824, "Interface in"=w825) -> ("error out"=w821:errorcluster, "Previous CCD Config"=w823:T6)  [unwired: 7 in, 1 out]
              n388 = Unbundle By Name(w823) -> ("FINAL_LINE"=w822:u16)
              n389 = Number To Fractional String(number=w822) -> (F-format string=w828:string)  [unwired: 3 in]
            }
            frame "INITIAL_COLUMN" {
              n390 = Unbundle By Name(w838) -> ("Simulated_CCD_Camera.lvclass"=w836:refnum<class "Simulated_CCD_Camera.lvclass">)
              n391 = call "Read Interface.lvclass.vi"("error in (no error)"=w835, "Simulated_CCD_Camera in"=w836) -> ("error out"=w833:errorcluster, "Interface.lvclass"=w834:refnum<class "Interface.lvclass">)  [unwired: 7 in, 1 out]
              n392 = call "Read Previous CCD Config.vi"("error in (no error)"=w833, "Interface in"=w834) -> ("error out"=w830:errorcluster, "Previous CCD Config"=w832:T6)  [unwired: 7 in, 1 out]
              n393 = Unbundle By Name(w832) -> ("INITIAL_COLUMN"=w831:u16)
              n394 = Number To Fractional String(number=w831) -> (F-format string=w837:string)  [unwired: 3 in]
            }
            frame "INITIAL_LINE" {
              n395 = Unbundle By Name(w847) -> ("Simulated_CCD_Camera.lvclass"=w845:refnum<class "Simulated_CCD_Camera.lvclass">)
              n396 = call "Read Interface.lvclass.vi"("error in (no error)"=w844, "Simulated_CCD_Camera in"=w845) -> ("error out"=w842:errorcluster, "Interface.lvclass"=w843:refnum<class "Interface.lvclass">)  [unwired: 7 in, 1 out]
              n397 = call "Read Previous CCD Config.vi"("error in (no error)"=w842, "Interface in"=w843) -> ("error out"=w839:errorcluster, "Previous CCD Config"=w841:T6)  [unwired: 7 in, 1 out]
              n398 = Unbundle By Name(w841) -> ("INITIAL_LINE"=w840:u16)
              n399 = Number To Fractional String(number=w840) -> (F-format string=w846:string)  [unwired: 3 in]
            }
            frame "COMMENT" {
              n400 = Unbundle By Name(w853) -> ("Save Image.lvclass"=w851:refnum<class "Save Image.lvclass">)
              n401 = call "Read Header parameters.vi"("error in (no error)"=w850, "Save Image in"=w851) -> ("error out"=w849:errorcluster, "Header parameters"=w852:T7)  [unwired: 7 in, 1 out]
              n402 = Unbundle By Name(w852) -> ("OBSTYPE"=w848:string)
            }
            frame "SUFFIX" {
              n403 = Unbundle By Name(w858) -> ("Save Image.lvclass"=w854:refnum<class "Save Image.lvclass">)
              n404 = call "Read Suffix image name.vi"("error in (no error)"=w855, "Save Image in"=w854) -> ("error out"=w857:errorcluster, "Suffix image name"=w856:string)  [unwired: 7 in, 1 out]
            }
            frame "OBSTYPE" {
              n405 = Unbundle By Name(w864) -> ("Save Image.lvclass"=w863:refnum<class "Save Image.lvclass">)
              n406 = call "Read Header parameters.vi"("error in (no error)"=w859, "Save Image in"=w863) -> ("error out"=w860:errorcluster, "Header parameters"=w862:T7)  [unwired: 7 in, 1 out]
              n407 = Unbundle By Name(w862) -> ("OBSTYPE"=w861:string)
            }
            frame "TEMP" {
              n408 = Unbundle By Name(w873) -> ("Simulated_CCD_Camera.lvclass"=w868:refnum<class "Simulated_CCD_Camera.lvclass">)
              n409 = call "Read Interface.lvclass.vi"("error in (no error)"=w867, "Simulated_CCD_Camera in"=w868) -> ("error out"=w871:errorcluster, "Interface.lvclass"=w869:refnum<class "Interface.lvclass">)  [unwired: 7 in, 1 out]
              n410 = call "Read Previous SET parameters.vi"("error in (no error)"=w871, "Interface in"=w869) -> ("error out"=w866:errorcluster, "Previous SET parameters"=w870:T8)  [unwired: 7 in, 1 out]
              n411 = Unbundle By Name(w870) -> ("TEMP"=w865:i32)
              n412 = Number To Decimal String(number=w865) -> (decimal integer string=w872:string)  [unwired: 1 in]
            }
            frame "SHUTTER_MODE" {
              n413 = Unbundle By Name(w882) -> ("Simulated_CCD_Camera.lvclass"=w877:refnum<class "Simulated_CCD_Camera.lvclass">)
              n414 = call "Read Interface.lvclass.vi"("error in (no error)"=w876, "Simulated_CCD_Camera in"=w877) -> ("error out"=w880:errorcluster, "Interface.lvclass"=w878:refnum<class "Interface.lvclass">)  [unwired: 7 in, 1 out]
              n415 = call "Read Previous CCD Config.vi"("error in (no error)"=w880, "Interface in"=w878) -> ("error out"=w875:errorcluster, "Previous CCD Config"=w879:T6)  [unwired: 7 in, 1 out]
              n416 = Unbundle By Name(w879) -> ("SHUTTER_MODE"=w874:T3)
              n417 = Number To Decimal String(number=w874) -> (decimal integer string=w881:string)  [unwired: 1 in]
            }
            frame "PREAMP" {
              n418 = Unbundle By Name(w891) -> ("Simulated_CCD_Camera.lvclass"=w886:refnum<class "Simulated_CCD_Camera.lvclass">)
              n419 = call "Read Interface.lvclass.vi"("error in (no error)"=w885, "Simulated_CCD_Camera in"=w886) -> ("error out"=w889:errorcluster, "Interface.lvclass"=w887:refnum<class "Interface.lvclass">)  [unwired: 7 in, 1 out]
              n420 = call "Read Previous CCD Config.vi"("error in (no error)"=w889, "Interface in"=w887) -> ("error out"=w884:errorcluster, "Previous CCD Config"=w888:T6)  [unwired: 7 in, 1 out]
              n421 = Unbundle By Name(w888) -> ("PREAMP"=w883:enum16{"Gain 1", "Gain 2"})
              n422 = Number To Decimal String(number=w883) -> (decimal integer string=w890:string)  [unwired: 1 in]
            }
            frame "#FRAMES" {
              n423 = Unbundle By Name(w900) -> ("Simulated_CCD_Camera.lvclass"=w898:refnum<class "Simulated_CCD_Camera.lvclass">)
              n424 = call "Read Interface.lvclass.vi"("error in (no error)"=w897, "Simulated_CCD_Camera in"=w898) -> ("error out"=w894:errorcluster, "Interface.lvclass"=w895:refnum<class "Interface.lvclass">)  [unwired: 7 in, 1 out]
              n425 = call "Read Previous SET parameters.vi"("error in (no error)"=w894, "Interface in"=w895) -> ("error out"=w893:errorcluster, "Previous SET parameters"=w896:T8)  [unwired: 7 in, 1 out]
              n426 = Unbundle By Name(w896) -> ("#FRAMES"=w892:u32)
              n427 = Number To Decimal String(number=w892) -> (decimal integer string=w899:string)  [unwired: 1 in]
            }
            frame "#CUBES" {
              n428 = Unbundle By Name(w909) -> ("Simulated_CCD_Camera.lvclass"=w907:refnum<class "Simulated_CCD_Camera.lvclass">)
              n429 = call "Read Interface.lvclass.vi"("error in (no error)"=w906, "Simulated_CCD_Camera in"=w907) -> ("error out"=w903:errorcluster, "Interface.lvclass"=w904:refnum<class "Interface.lvclass">)  [unwired: 7 in, 1 out]
              n430 = call "Read Previous SET parameters.vi"("error in (no error)"=w903, "Interface in"=w904) -> ("error out"=w901:errorcluster, "Previous SET parameters"=w905:T8)  [unwired: 7 in, 1 out]
              n431 = Unbundle By Name(w905) -> ("#CUBES"=w902:u32)
              n432 = Number To Decimal String(number=w902) -> (decimal integer string=w908:string)  [unwired: 1 in]
            }
          }
          n433 = Unbundle By Name(w741) -> ("RxTx.lvclass"=w743:refnum<class "RxTx.lvclass">)
          n434 = call "Send TX Message.vi"("error in (no error)"=w740, "element"=w739, "RxTx in"=w743) -> ("error out"=w733:errorcluster, "RxTx out"=w742:refnum<class "RxTx.lvclass">)  [unwired: 7 in]
          n435 = Bundle By Name(cluster=w741, "RxTx.lvclass"=w742) -> (w732:refnum<class "Channel.lvclass">)
          n436 = Unbundle By Name(w732) -> ("State Machine.lvclass"=w734:refnum<class "State Machine.lvclass">)
          n437 = call-dynamic "Write State.vi"("error in (no error)"=w733, "State"="False", "State Machine in"=w734) -> ("error out"=w730:errorcluster, "State Machine out"=w736:refnum<class "State Machine.lvclass">)  [unwired: 7 in]
          n438 = Bundle By Name(cluster=w732, "State Machine.lvclass"=w736) -> (w731:refnum<class "Channel.lvclass">)
        }
        frame "INIT_DEACTIVATED" {
          n439 = Unbundle By Name(w925) -> ("Simulated_CCD_Camera.lvclass"=w926:refnum<class "Simulated_CCD_Camera.lvclass">, "Save Image.lvclass"=w913:refnum<class "Save Image.lvclass">)
          n440 = call "Read Header parameters.vi"("error in (no error)"=w912, "Save Image in"=w913) -> ("error out"=w910:errorcluster, "Header parameters"=w914:T7)  [unwired: 7 in, 1 out]
          n441 = Unbundle By Name(w914) -> ("CHANNEL"=w911:u16)
          n442 = call-dynamic "Initialize Camera.vi"("error in (no error)"=w910, "channel"=w911, "CCDCamera in"=w926) -> ("error out"=w930:errorcluster, "CCDCamera out"=w931:refnum<class "Simulated_CCD_Camera.lvclass">)  [unwired: 7 in]
          n443 = call-dynamic "Standard Setup.vi"("error in (no error)"=w930, "CCDCamera in"=w931) -> ("error out"=w927:errorcluster, "CCDCamera out"=w928:refnum<class "Simulated_CCD_Camera.lvclass">)  [unwired: 8 in]
          n444 = call-dynamic "Set Camera Configuration.vi"("error in (no error)"=w927, "CCDCamera in"=w928) -> ("error out"=w920:errorcluster, "CCDCamera out"=w929:refnum<class "Simulated_CCD_Camera.lvclass">)  [unwired: 8 in]
          n445 = Bundle By Name(cluster=w925, "Simulated_CCD_Camera.lvclass"=w929) -> (w921:refnum<class "Channel.lvclass">)
          n446 = Unbundle By Name(w921) -> ("Save Image.lvclass"=w924:refnum<class "Save Image.lvclass">)
          n447 = call "Read Header parameters.vi"("error in (no error)"=w920, "Save Image in"=w924) -> ("error out"=w919:errorcluster, "Header parameters"=w917:T7, "Save Image out"=w923:refnum<class "Save Image.lvclass">)  [unwired: 7 in]
          n448 = Bundle By Name(cluster=w917, "NIGHTDIR"="E:\\images\\today") -> (w916:T7)
          n449 = call "Write Header parameters.vi"("error in (no error)"=w919, "Header parameters"=w916, "Save Image in"=w923) -> ("error out"=w918:errorcluster, "Save Image out"=w922:refnum<class "Save Image.lvclass">)  [unwired: 7 in]
          n450 = Bundle By Name(cluster=w921, "Save Image.lvclass"=w922) -> (w937:refnum<class "Channel.lvclass">)
          n451 = Unbundle By Name(w937) -> ("State Machine.lvclass"=w934:refnum<class "State Machine.lvclass">)
          n452 = call-dynamic "Write State.vi"("error in (no error)"=w918, "State"="False", "State Machine in"=w934) -> ("error out"=w932:errorcluster, "State Machine out"=w936:refnum<class "State Machine.lvclass">)  [unwired: 7 in]
          n453 = Bundle By Name(cluster=w937, "State Machine.lvclass"=w936) -> (w933:refnum<class "Channel.lvclass">)
        }
        frame "RESTART_COMMUNICATION" {
          n454 = Unbundle By Name(w944) -> ("State Machine.lvclass"=w946:refnum<class "State Machine.lvclass">)
          n455 = call "Verify Timer.vi"("error in (no error)"=w945, "State Machine in"=w946) -> ("error out"=w942:errorcluster, "time out"=w941:bool, "State Machine out"=w943:refnum<class "State Machine.lvclass">)  [unwired: 7 in]
          n456 = Bundle By Name(cluster=w944, "State Machine.lvclass"=w943) -> (w940:refnum<class "Channel.lvclass">)
          n457 = case shown="True" w941 {
            tunnel: w942 -> [w947 w951]
            tunnel: w940 -> [w948 w963]
            tunnel: [w948 w954] -> w939
            tunnel: [w947 w958] -> w938
            frame False {
            }
            frame True {
              n458 = Unbundle By Name(w963) -> ("Simulated_CCD_Camera.lvclass"=w957:refnum<class "Simulated_CCD_Camera.lvclass">, "Save Image.lvclass"=w952:refnum<class "Save Image.lvclass">)
              n459 = call "Read Header parameters.vi"("error in (no error)"=w951, "Save Image in"=w952) -> ("error out"=w949:errorcluster, "Header parameters"=w953:T7)  [unwired: 7 in, 1 out]
              n460 = Unbundle By Name(w953) -> ("CHANNEL"=w950:u16)
              n461 = call-dynamic "Initialize Camera.vi"("error in (no error)"=w949, "channel"=w950, "CCDCamera in"=w957) -> ("error out"=w968:errorcluster, "CCDCamera out"=w969:refnum<class "Simulated_CCD_Camera.lvclass">)  [unwired: 7 in]
              n462 = call "Read Interface.lvclass.vi"("error in (no error)"=w968, "Simulated_CCD_Camera in"=w969) -> ("error out"=w966:errorcluster, "Interface.lvclass"=w967:refnum<class "Interface.lvclass">, "Simulated_CCD_Camera out"=w955:refnum<class "Simulated_CCD_Camera.lvclass">)  [unwired: 7 in]
              n463 = call "Read Camera Status.vi"("error in (no error)"=w966, "Interface in"=w967) -> ("error out"=w956:errorcluster, "Camera Status"=w965:T2)  [unwired: 7 in, 1 out]
              n464 = Bundle By Name(cluster=w963, "Simulated_CCD_Camera.lvclass"=w955) -> (w960:refnum<class "Channel.lvclass">)
              n465 = Unbundle By Name(w965) -> ("CCD_ON_OFF"=w964:bool)
              n466 = case shown="True" w964 {
                tunnel: ["RESTART_COMMUNICATION" "False"] -> w961
                frame False {
                }
                frame True {
                }
              }
              n467 = Unbundle By Name(w960) -> ("State Machine.lvclass"=w962:refnum<class "State Machine.lvclass">)
              n468 = call-dynamic "Write State.vi"("error in (no error)"=w956, "State"=w961, "State Machine in"=w962) -> ("error out"=w958:errorcluster, "State Machine out"=w959:refnum<class "State Machine.lvclass">)  [unwired: 7 in]
              n469 = Bundle By Name(cluster=w960, "State Machine.lvclass"=w959) -> (w954:refnum<class "Channel.lvclass">)
            }
          }
        }
      }
    }
    frame Error {
    }
  }
  "error out" <- w3
  "Channel out" <- w1
